vi "MoD Main-Optimize - HPLCv2 SnAr.vi"() -> ()   [LabVIEW 2015]
uses:
  <vilib>/silver_ctls/ArrayMatrixCluster/Real Matrix NI_Silver.ctl
  <vilib>/ni845x/ni845x.llb/ni845xControl.ctl
  <vilib>/MakerHub/LINX/Public/Peripherals/Analog/Analog Read 1 Chan.vi
  <vilib>/MakerHub/LINX/Public/Peripherals/Analog/Analog Read N Chans.vi
  <vilib>/MakerHub/LINX/Public/Peripherals/Digital/Digital Write 1 Chan.vi
  <vilib>/MakerHub/LINX/Private/Local IO/LinxAnalogRead.vi
  <vilib>/MakerHub/LINX/Public/Utilities/Check Channel.vi
  <vilib>/MakerHub/LINX/Public/Peripherals/Digital/Digital Write N Chans.vi
  <vilib>/MakerHub/LINX/Private/Local IO/LinxDigitalWrite.vi
  <vilib>/addons/control/pid/pid.llb/PID Control Input Filter (DBL).vi
  <vilib>/MakerHub/LINX/Private/Utilties/Generate Error.vi
  <vilib>/addons/control/pid/autopid.llb/PID Online Autotuning (Relay Feedback).vi
  <vilib>/Analysis/Matrix/Numeric/Conversions/Array To Matrix - RA2.vi
  <vilib>/ni845x/ni845x.llb/NI-845x Close Device Reference.vi
  <vilib>/addons/control/pid/NI_PID_autopid.lvlib
  <vilib>/addons/control/pid/NI_PID_pid.lvlib
  <vilib>/Analysis/Matrix/NI_Matrix.lvlib
  <vilib>/MakerHub/LINX/LMH-LINX.lvlib
  <instrlib>/Harvard Apparatus PHD Ultra Series/Harvard Apparatus PHD Ultra Series.lvlib
panel:
  out "running?":bool=TRUE
  out "new_reactor_volume":bool[](array[boolean])
  out "new_reactor_length":bool[](array[boolean])
  out "Phase_Sensor_voltage":dbl
  out "P_tot":dbl
  out "pause for ms":bool=TRUE
  out "stop_xl_write":bool=TRUE
  out "Num_exp_till_pause":i32
  out "Syringe_pump?":bool=TRUE
  out "System Error":bool=TRUE
  out "error out":errorcluster
  out "Pump setpoint(ul/min) 6":dbl format="%#_13g"
  out "Pump setpoint(ul/min) 5":dbl format="%#_13g"
  out "Pump setpoint(ul/min) 4":dbl format="%#_13g"
  out "Pump setpoint(ul/min) 3":dbl format="%#_13g"
  out "Pump setpoint(ul/min) 2":dbl format="%#_13g"
  out "Pump setpoint(ul/min) 1":dbl format="%#_13g"
  out "Volume (ul) 5":dbl format="%#_13g"
  out "Volume (ul) 4":dbl format="%#_13g"
  out "Volume (ul) 3":dbl format="%#_13g"
  out "Volume (ul) 2":dbl format="%#_13g"
  out "Volume (ul) 1":dbl format="%#_13g"
  in  "tau 5":dbl format="%#_13g"
  out "tau 4":dbl format="%#_13g"
  out "tau 3":dbl format="%#_13g"
  out "tau 2":dbl format="%#_13g"
  out "tau 1":dbl format="%#_13g"
  out "Reactor Length":dbl format="%#_13g"
  out "Flowrate Sensor 2":dbl format="%#_13g"
  out "Flowrate Sensor 1":dbl format="%#_13g"
  out "Pressure 2":dbl format="%#_13g"
  out "Pressure 1":dbl format="%#_13g"
  out "Temperature Control 5":bool=TRUE
  out "Temperature Control 4":bool=TRUE
  out "Temperature Control 3":bool=TRUE
  out "Temperature Control 2":bool=TRUE
  out "Temperature Control 1":bool=TRUE
  out "Temperature SP 5":dbl format="%#_g'C"
  out "Temperature SP 4":dbl format="%#_g'C"
  out "Temperature SP 3":dbl format="%#_g'C"
  out "Temperature SP 2":dbl format="%#_g'C"
  out "Temperature SP 1":dbl format="%#_g'C"
  in  "Bay Temperature 5":dbl
  in  "SSR Duration 5":dbl
  in  "SSR Duration 4":dbl
  in  "SSR Duration 3":dbl
  in  "SSR Duration 2":dbl
  in  "SSR Duration 1":dbl
  in  "Total Product Amount":dbl=1.0 format="%#_gml"
  out "Setup Error":bool=TRUE
  out "Error Message":string
  out "ID CTR":i32
  in  "Tab Control":T1(tab)
  out "Reagent pic 5":picture
  in  "reagent name 5":string
  out "Reagent Pic 4":picture
  in  "reagent name 4":string="DMF"
  out "Reagent Pic 3":picture
  in  "reagent  name 3":string="tributylamine"
  in  "Product name":string
  in  "reagent name 1":string="2-chloronitrobenzene"
  out "Reagent Pic 1":picture
  in  "Vr5":dbl format="%#_guL"
  in  "Vr4":dbl format="%#_guL"
  in  "Vr3":dbl format="%#_guL"
  in  "Vr2":dbl format="%#_guL"
  in  "Vr1":dbl format="%#_guL"
  in  "System decide help Button":bool
  in  "Reaction Scheme Confirm":bool
  in  "Synthesis Route Array":string[][](array[string])=[["2-chloronitrobenzene", "1.0", "PhB(OH)2", "", "", ""], ["1,2,3,4-tetrahydroquinoline", "1.0", "-", "-", "-", "-"], ["tributylamine", "1.0", "-", "-", "-", "-"], ["DMF", "8", "-", "-", "-", "-"]]
  in  "System decide help Button 2":bool
  out "Setup Confirm":bool=TRUE
  in  "BAY 1":u16(ring) items=["               Bypass", "         Heated Reactor", "    Small Heated Reator", "         Cooled Reactor", "      Packed Bed Reactor", "          Photo Reactor", "             Separator"]
  in  "BAY 5":u16(ring) items=["               Bypass", "         Heated Reactor", "    Small Heated Reactor", "         Cooled Reactor", "     Packed Bed Reactor", "         Photo Reactor", "             Separator"]
  in  "BAY 4":u16(ring)=1 items=["                Bypass", "         Heated Reactor", "    Small Heated Reactor", "         Cooled Reactor", "     Packed Bed Reactor", "         Photo Reactor", "             Separator"]
  in  "BAY 3":u16(ring) items=["               Bypass", "         Heated Reactor", "    Small Heated Reactor", "         Cooled Reactor", "     Packed Bed Reactor", "          Photo Reactor", "             Separator"]
  in  "BAY 2":u16(ring) items=["               Bypass", "         Heated Reactor", "    Small Heated Reactor", "         Cooled Reactor", "      Packed Bed Reactor", "          Photo Reactor", "             Separator"]
  out "Reagent Pic 2":picture
  out "Product Pic":picture
  in  "reagent name 2":string="1,2,3,4-tetrahydroquinoline"
  in  "reagent name 6":string
  out "Reagent Pic 6":picture
  in  "System Parameters Help Button":bool
  out "Setup Confirm 2":bool
  in  "System Parameters Confirm Button":bool
  in  "Bay Parameters":T2={"Bay 1 "={"Pump 1 Flowrate"=0.0, "optimize_temp"=FALSE, "optimize_tau"=TRUE, "Run at set flowrate"=FALSE, "Pump 2 Flowrate"=0.0, "Temperature Params"=[40.0, 100.0, 100.0], "pump params 1"=[21.0, 214.0, 325.0], "pump params 2"=[21.0, 214.0, 325.0], "Temperature"=0.0, "Run at set temperature"=FALSE}, "Bay 2 "={"Pump 3 Flowrate"=0.0, "optimize_temp"=FALSE, "optimize_tau"=FALSE, "Run at set flowrate"=TRUE, "Temperature Params"=[40.0, 100.0, 100.0], "Resisdence time params"=[65.0, 650.0, 650.0], "pump_at_ratio"=FALSE, "pump_num_ratio"=1.0, "Temperature"=0.0, "Run at set temperature"=FALSE}, "Bay 3 "={"Pump 4 Flowrate"=100.0, "optimize_temp"=FALSE, "optimize_tau"=TRUE, "Run at set flowrate"=FALSE, "Temperature Params"=[40.0, 100.0, 100.0], "Resisdence time params"=[21.0, 214.0, 0.0], "pump_at_ratio"=FALSE, "pump_num_ratio"=0.0, "Temperature "=0.0, "Run at set temperature"=FALSE}, "Bay 4 "={"Pump 5 Flowrate"=40.0, "Run at set flowrate"=FALSE, "optimize_temp"=TRUE, "optimize_tau"=FALSE, "Resisdence time params"=[0.0, 36.0, 225.0], "Temperature Params"=[40.0, 100.0, 80.0], "pump_at_ratio"=FALSE, "pump_num_ratio"=0.0, "Temperature"=0.0, "Run at set temperature"=FALSE}, "Bay 5 "={"Pump 6 Flowrate"=0.0, "Run at set flowrate"=FALSE, "optimize_temp"=FALSE, "optimize_tau"=FALSE, "Resisdence time params"=[0.0, 0.0, 0.0], "Temperature Params"=[0.0, 0.0, 0.0], "pump_at_ratio"=FALSE, "pump_num_ratio"=0.2, "Temperature"=0.0, "Run at set temperature"=FALSE}, "Excel File Name"="C:\\Users\\HPLC\\Dropbox (MIT)\\MoD Files\\Data\\SNAR_043017", "hplc File Name"="C:\\Chem32\\1\\Data\\MOD", "Matlab File"="C:\\Users\\HPLC\\Dropbox (MIT)\\MoD Files\\Data\\SNAR_043017", "Syringe for Pump 2?"=TRUE, "Num_conditons_per_wait"=1.0, "Continue from previous optimization?"=FALSE, "Total Number of Experiments 2"=33.0, "Hplc Wait time(min)"=14.0, "increas_decrease_hplc_peak"=FALSE, "Internal Standard?"=TRUE, "ISTD start"=10.0, "ISTD end"=14.0, "hplc_start"=2.3, "hplc_end"=2.8, "throughput_yield"=FALSE} {"Hplc Wait time(min)" format="%#_13g"; "Bay 5"."Temperature Params" format="%#_g'C"; "Bay 4"."Temperature Params" format="%#_g'C"; "Bay 3"."Temperature Params" format="%#_g'C"; "Bay 2"."Temperature Params" format="%#_g'C"; "Bay 1"."Temperature Params" format="%#_g'C"}
  out "System Confirm Not Clicked":string
  out "best_exp_num":dbl=1.0
  out "temperature_best":dbl[](array[numeric])
  out "Flowrates(ul/min)_best":dbl[](array[numeric])
  out "System Status":u16(ring)=2 caption="Sy" items=["System  Error", "System Running", "System Standby"]
  out "Current Experiment":dbl=1.0
  out "Total Number of Experiments":dbl=33.0
  out "Phase Sensor Chart":T3(graph)
  out "HPLC Analysis":bool
  out "Equlibrating Temperature":bool
  out "Flushing System":bool
  out "Calculate condition":bool
  out "Temperature 5":dbl format="%#_g'C"
  out "Temperature 4":dbl format="%#_g'C"
  out "Temperature 3":dbl format="%#_g'C"
  out "Temperature 2":dbl format="%#_g'C"
  out "Temperature 1":dbl format="%#_g'C"
  out "Flowrate Chart":T4(graph)
  out "Teperature Chart":T3(graph)
  out "Pump Setpoints Chart":T3(graph)
  out "Pressure Chart":T3(graph)
  out "Optimization_loop_index":i32
  out "curr_wait_time":dbl
  out "total_flush_time":dbl
  out "Temp SS? 5":bool=TRUE
  out "Temp SS? 4":bool=TRUE
  out "Temp SS? 3":bool=TRUE
  out "Temp SS? 2":bool=TRUE
  out "Temp SS? 1":bool=TRUE
  out "System Flushed?":bool
  out "stop_button clicked":bool
  out "experiment history":T5
  in  "Number of System Flushes per condtion":dbl=2.5
  in  "calculate volume 3":bool
  in  "calculate volume 2":bool
  in  "calculate volume 1":bool
  in  "calculate volume 4":bool
  in  "calculate volume 5":bool
  in  "Extra system dead volume":dbl format="%#_gul"
  in  "new reactor length? 1":bool
  in  "tube_length(in)":dbl[](array[numeric])=[188.0, 188.0, 10.0, 10.0, 10.0]
  out "Pause Before Analysis":bool
  out "Chiller COMM Port":bool
  out "Arduino COMM Port 2":bool
  out "Temperature Sensor COMM Port":bool
  out "Flow Rate":bool
  out "Pressure":bool
  out "Pump COMM Port":bool
  in  "COMM Port :: Milligat Pumps":refnum<visa-resource-name>="COM10"
  in  "Arduino COMM Port":refnum<visa-resource-name>="COM3"
  in  "Sample Valve COMM::Port":refnum<visa-resource-name>="COM6"
  in  "COMM Port:: Harvard Syringe Pump":refnum<visa-resource-name>="COM5"
  in  "tube_id(in)":enum16{".01", ".02", ".03", ".04"}[](array[ring])=[enum.".03", enum.".03", enum.".03", enum.".03", enum.".03"]
  out "Total System Resisdence Time(min)":dbl
  in  "Debug_run_button":bool
  in  "new reactor length? 2":bool
  in  "new reactor length? 3":bool
  in  "new reactor length? 4":bool
  in  "new reactor length? 5":bool
  in  "IR Sensor Device":T6="USB0::0x3923::0x7514::01B3FF21::RAW"
  out "Stop":bool=TRUE
  in  "Run_Stop_cluster":T7
  # "Molecules on Demand"
  # "Synthetic Route"
  # "5"
  # "6"
  # "4"
  # "Product"
  # "1"
  # "2"
  # "3"
  # "Reagent List"
  # "Concentration(M)"
  # "Molecule"
  # "1"
  # "1"
  # "2"
  # "2"
  # "3"
  # "3"
  # "4"
  # "4"
  # "5"
  # "6"
  # "5"
  # "6"
  # "Product"
  # "Reactor Volume:"
  # "Optimization Parameters"
  # "Pause after"
  # "Experiments"
  # "Optimize for"
  # "to"
  # "of HPLC Peak from"
  # "from"
  # "to"
  # "min"
  # "min"
  # "HPLC runtime"
  # "# Iterations"
  # "Reporting"
  # "Excel Output File Name"
  # "HPLC File Path"
  # "MATLAB File Path"
  # "Temperature"
  # "Flowrate(ul/min)"
  # "Lower Bound"
  # "Upper Bound"
  # "Optimize?"
  # "-or-"
  # "Run at"
  # "times incoming flow"
  # "Setpoint"
  # "Temperature"
  # "Flowrate(ul/min)"
  # "Lower Bound"
  # "Upper Bound"
  # "Optimize?"
  # "-or-"
  # "Run at"
  # "times incoming flow"
  # "Setpoint"
  # "Temperature"
  # "Flowrate(ul/min)"
  # "Lower Bound"
  # "Upper Bound"
  # "Optimize?"
  # "-or-"
  # "Run at"
  # "times incoming flow"
  # "Setpoint"
  # "Temperature"
  # "Flowrate 3 (ul/min)"
  # "Lower Bound"
  # "Upper Bound"
  # "Optimize?"
  # "-or-"
  # "Run at"
  # "times incoming flow"
  # "Setpoint"
  # "Temperature"
  # "Flowrate 1(ul/min)"
  # "Flowrate 2(ul/min)"
  # "Lower Bound"
  # "Upper Bound"
  # "Optimize?"
  # "Setpoint"
  # "Pressure (psi)"
  # "System Status"
  # "Temperature('C)"
  # "BAY"
  # "1"
  # "2"
  # "3"
  # "4"
  # "5"
  # "Pump Flowrate Setpoint(ul/min)"
  # "Flowrate (ul/min)"
  # "Phase Sensor"
  # "Current Experiment"
  # "Temperature('C)"
  # "Flowrate(ul/min)"
  # "Exp"
  # "Current Best Condition"
  # "Time to reach steady state:"
  # "Current Wait Time:"
  # "Experimental Steps"
  # "Calculated new conditions"
  # "Flushed System"
  # "Analyzed HPLC"
  # "Equilibrated Temperature"
  # "Tube Length (cm)"
  # "Bay"
  # "Tube ID (in)"
  # "Calculate Volume"
  # "Use new tube length"
  # "1."
  # "2."
  # "3."
  # "4."
  # "5."
  # "Reactor Lengths\n*Heated Reactor - 188cm * Small Reactor - 99cm * Bypass - 10cm * Separator - *"
  # "All Experimental Data"
  # "P1"
  # "P2"
  # "P3"
  # "P4"
  # "P5"
  # "P6"
  # "T1"
  # "T2"
  # "T3"
  # "T4"
  # "T5"
  # "Obj_fun"
  # "HPLC_Data"
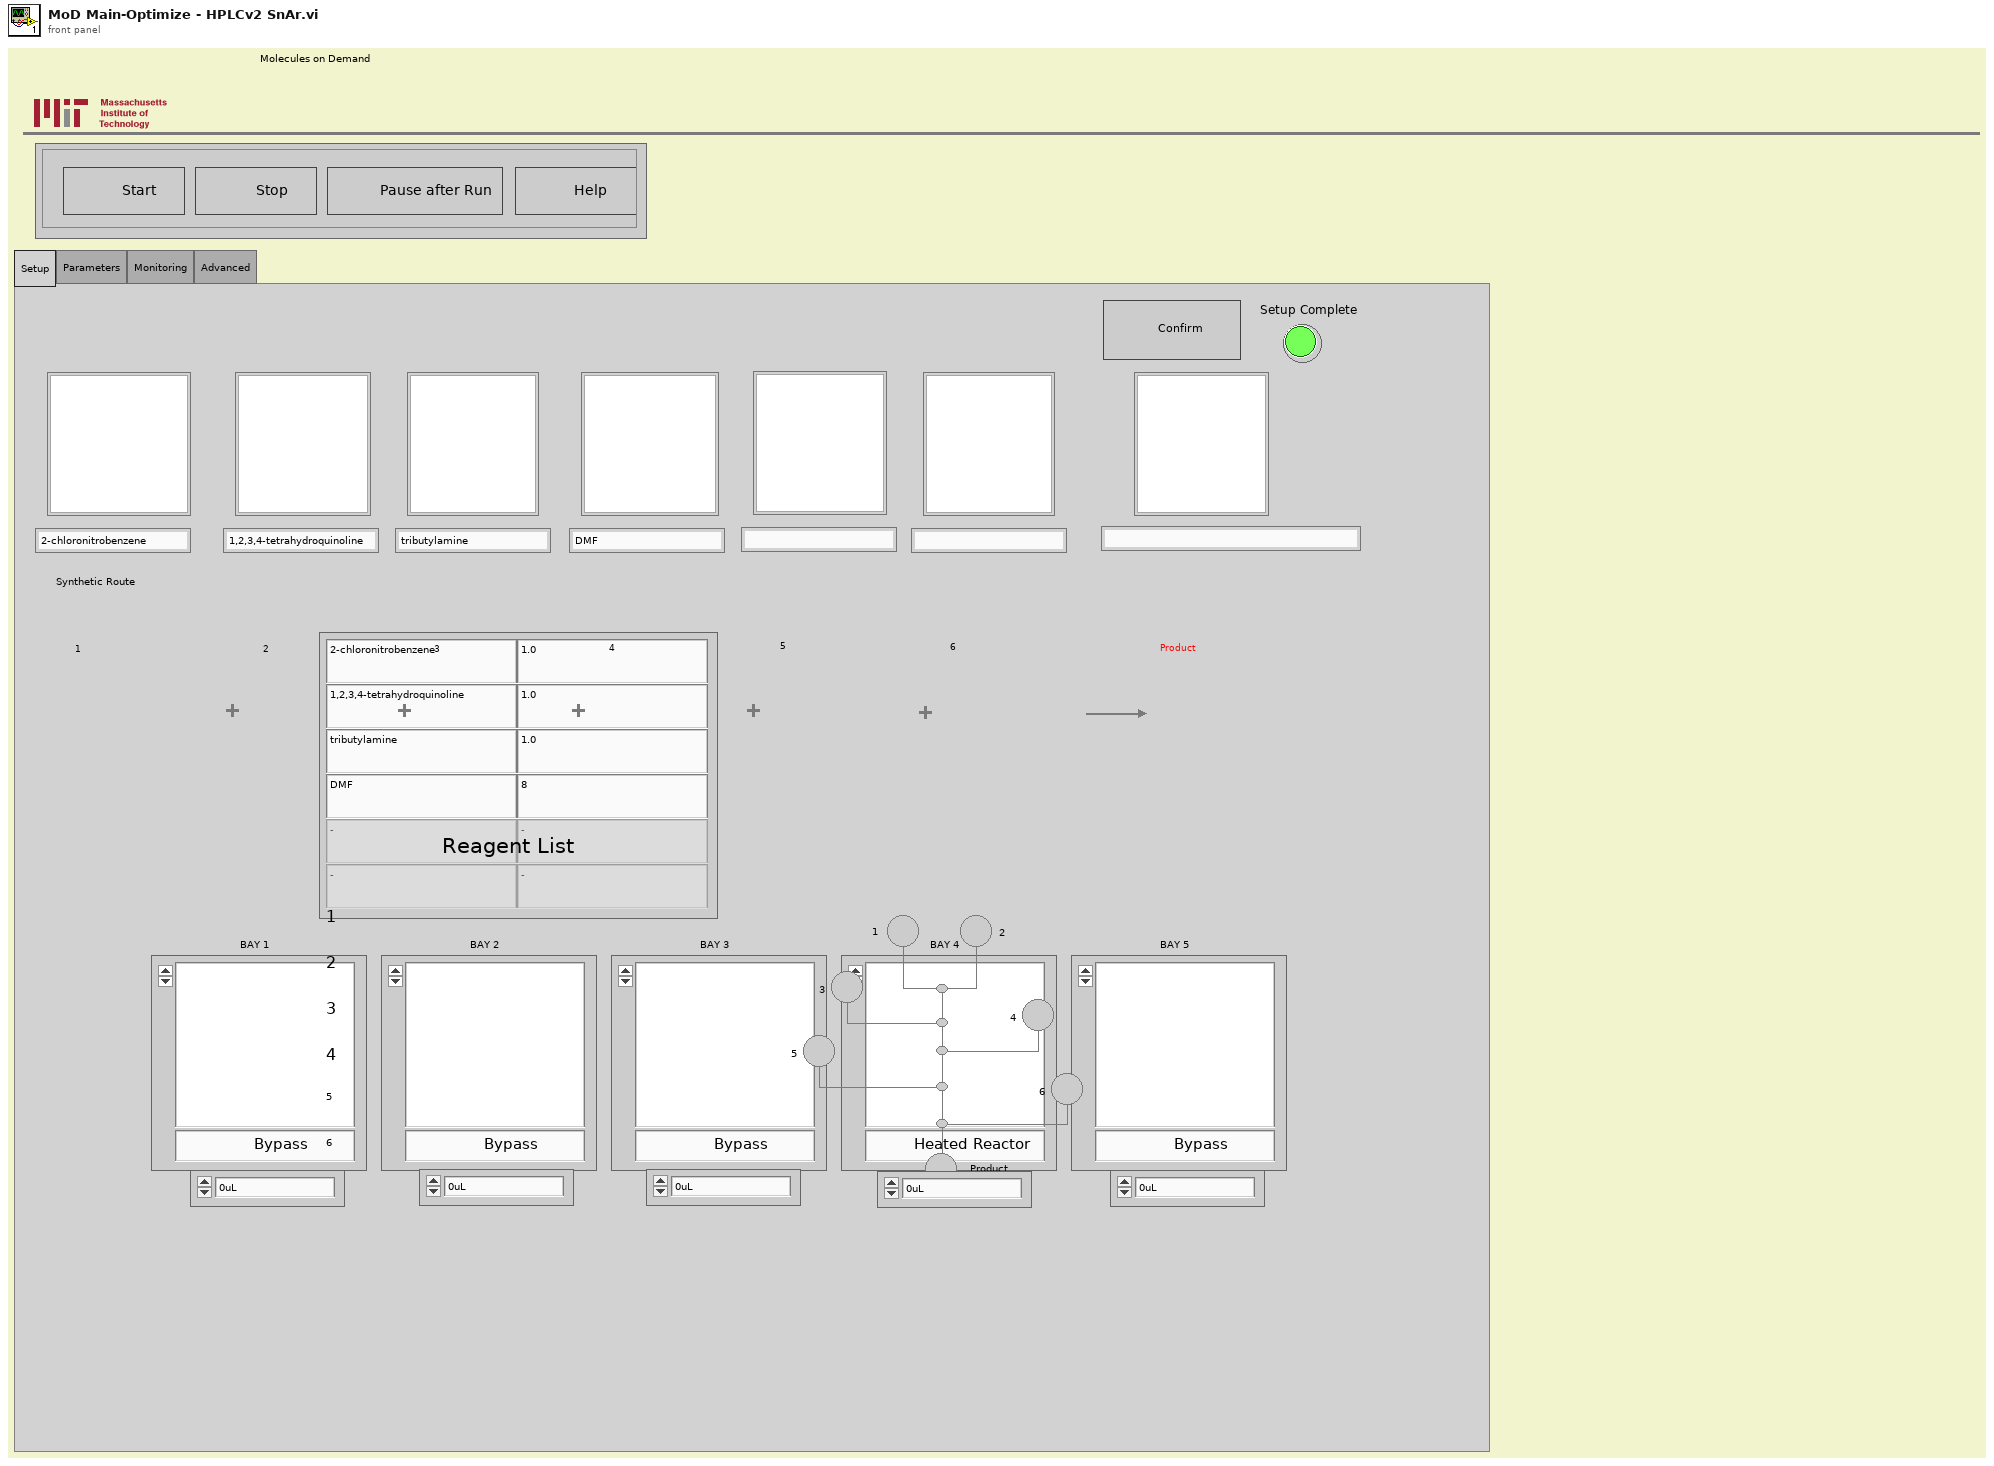
[diagram p1: front panel]
types:
  T1 = enum32{"Setup", "Parameters", "Monitoring", "Advanced"}
  T2 = cluster{"Bay 1 ":cluster{"Pump 1 Flowrate":dbl, "optimize_temp":bool, "optimize_tau":bool, "Run at set flowrate":bool, "Pump 2 Flowrate":dbl, "Temperature Params":dbl[], "pump params 1":dbl[], "pump params 2":dbl[], "Temperature":dbl, "Run at set temperature":bool}, "Bay 2 ":cluster{"Pump 3 Flowrate":dbl, "optimize_temp":bool, "optimize_tau":bool, "Run at set flowrate":bool, "Temperature Params":dbl[], "Resisdence time params":dbl[], "pump_at_ratio":bool, "pump_num_ratio":dbl, "Temperature":dbl, "Run at set temperature":bool}, "Bay 3 ":cluster{"Pump 4 Flowrate":dbl, "optimize_temp":bool, "optimize_tau":bool, "Run at set flowrate":bool, "Temperature Params":dbl[], "Resisdence time params":dbl[], "pump_at_ratio":bool, "pump_num_ratio":dbl, "Temperature ":dbl, "Run at set temperature":bool}, "Bay 4 ":cluster{"Pump 5 Flowrate":dbl, "Run at set flowrate":bool, "optimize_temp":bool, "optimize_tau":bool, "Resisdence time params":dbl[], "Temperature Params":dbl[], "pump_at_ratio":bool, "pump_num_ratio":dbl, "Temperature":dbl, "Run at set temperature":bool}, "Bay 5 ":cluster{"Pump 6 Flowrate":dbl, "Run at set flowrate":bool, "optimize_temp":bool, "optimize_tau":bool, "Resisdence time params":dbl[], "Temperature Params":dbl[], "pump_at_ratio":bool, "pump_num_ratio":dbl, "Temperature":dbl, "Run at set temperature":bool}, "Excel File Name":string, "hplc File Name":string, "Matlab File":string, "Syringe for Pump 2?":bool, "Num_conditons_per_wait":dbl, "Continue from previous optimization?":bool, "Total Number of Experiments 2":dbl, "Hplc Wait time(min)":dbl, "increas_decrease_hplc_peak":bool, "Internal Standard?":bool, "ISTD start":dbl, "ISTD end":dbl, "hplc_start":dbl, "hplc_end":dbl, "throughput_yield":bool}
  T3 = cluster{"[0]":dbl, "[1]":dbl, "[2]":dbl, "[3]":dbl, "[4]":dbl, "[5]":dbl, "[6]":dbl, "[7]":dbl, "[8]":dbl}
  T4 = cluster{"[0]":i32, "[1]":i32, "[2]":i32, "[3]":i32, "[4]":i32, "[5]":i32, "[6]":i32, "[7]":i32, "[8]":i32}
  T5 = typedef "Real Matrix NI_Silver.ctl" = dbl[][]
  T6 = typedef "ni845xControl.ctl" = refnum<k21>
  T7 = cluster{"Stop":bool, "Run":bool, "Stop Run Button":bool, "Help Button":bool}
  T8 = cluster{"Proportional gain Kc":dbl, "Integral time Ti (sec)":dbl, "Derivative time Ti (sec)":dbl}
  T9 = cluster{"type of controller":enum16{"P", "PI", "PID"}, "relay cycles":i32, "relay amplitude":dbl, "control specifications":enum16{"Fast", "Normal", "Slow"}, "PV noise level":dbl}
  T10 = typedef "LMH-LINX.lvlib/LINX Ref.ctl" = cluster{"IO":T11, "Interface":T12, "LINX Device Config":T13}
  T11 = typedef "LMH-LINX.lvlib/Platform.ctl" = enum16{"Remote", "Local"}
  T12 = typedef "LMH-LINX.lvlib/Interface.ctl" = enum16{"Serial", "TCP"}
  T13 = typedef "LMH-LINX.lvlib/Device.lvlib/LINX Device Config.ctl" = cluster{"Interface":T12, "COM Port":refnum<visa-resource-name>, "TCP Configuration":T14, "Device Family":u8, "Device ID":u8, "Device Name":string, "TCP Ref":refnum<k5>, "Channels":T15}
  T14 = typedef "LMH-LINX.lvlib/Device.lvlib/TCP Config.ctl" = cluster{"IP Address":string, "Port":u16}
  T15 = typedef "LMH-LINX.lvlib/Channels.ctl" = cluster{"DI":u8[], "DO":u8[], "AI":u8[], "AO":u8[], "PWM":u8[], "QE":u8[], "UART":u8[], "I2C 2":u8[], "SPI":u8[], "CAN":u8[], "Servo":u8[], "AI Ref (V)":dbl, "AI Resolution (Bits)":u8, "AO Ref (V)":dbl, "AO Resolution (Bits)":u8}
  T16 = typedef "imagedata.ctl" = cluster{"image type":i32, "image depth":i32, "image":u8[], "mask":u8[], "colors":u32[], "Rectangle":cluster{"left":i16, "top":i16, "right":i16, "bottom":i16}}
  T17 = cluster{"proportional gain (Kc)":dbl, "integral time (Ti, min)":dbl, "derivative time (Td, min)":dbl}
  T18 = typedef "NI_Matrix.lvlib/RealMatrix.ctl" = dbl[][]
  T19 = enum16{"Left Button", "Center Button", "Right Button", "Window Close"}
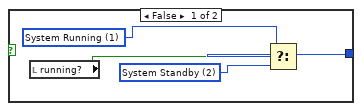
[diagram p3: hidden frame]
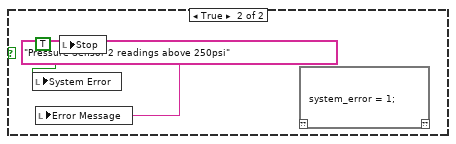
[diagram p4: hidden frame]
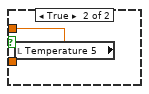
[diagram p6: hidden frame]
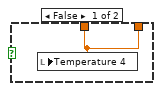
[diagram p7: hidden frame]
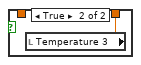
[diagram p8: hidden frame]
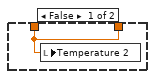
[diagram p9: hidden frame]
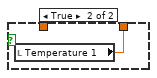
[diagram p10: hidden frame]
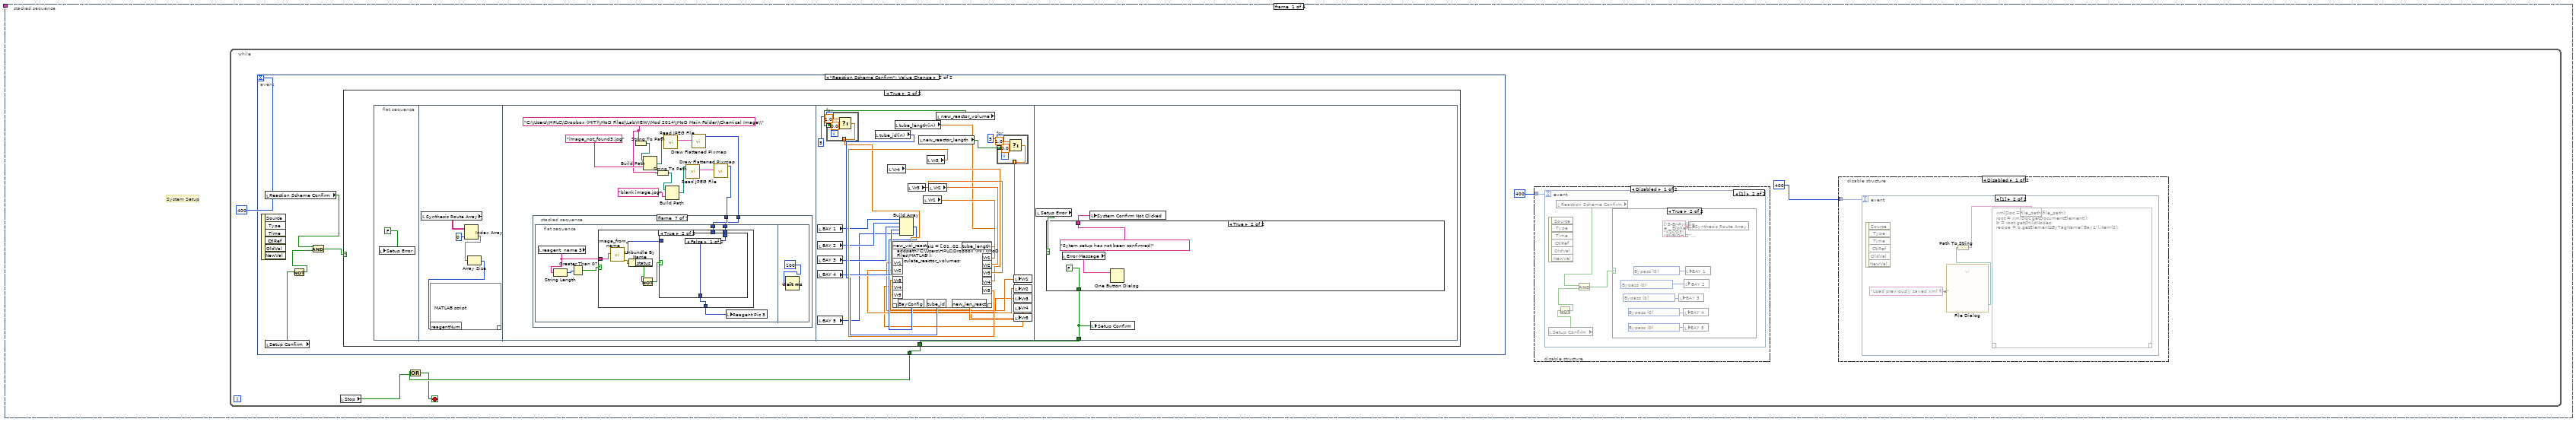
[diagram p11: hidden frame]
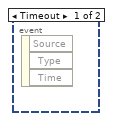
[diagram p12: hidden frame]
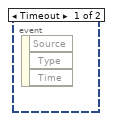
[diagram p14: hidden frame]
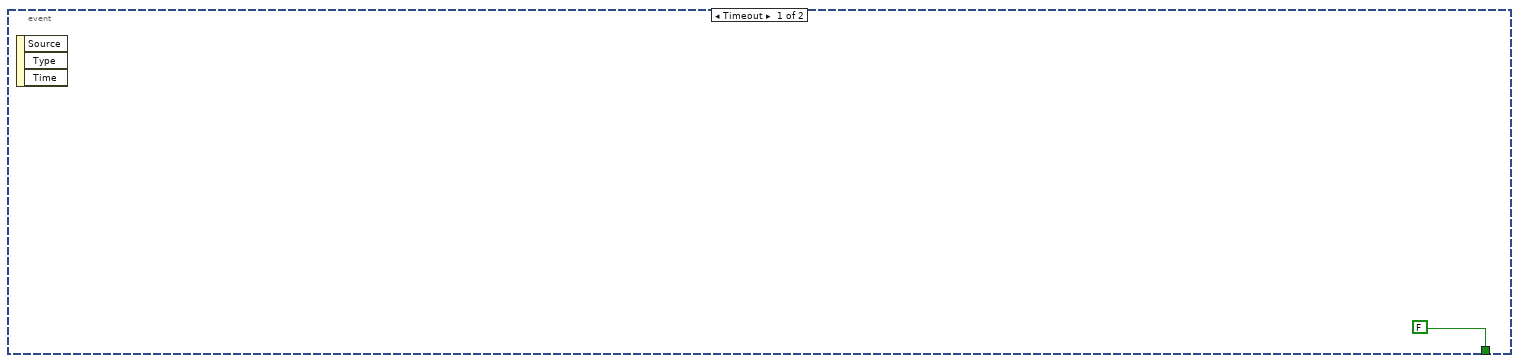
[diagram p17: hidden frame]
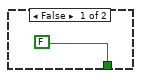
[diagram p18: hidden frame]
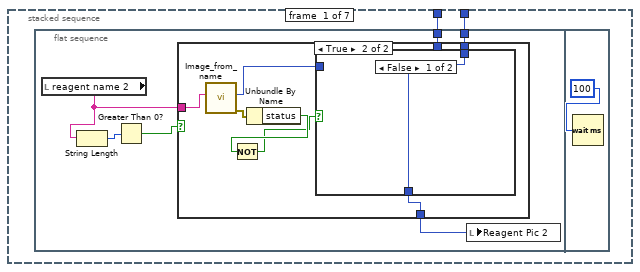
[diagram p19: hidden frame]
diagram:
  # "Assume User always uses the first bay first"
  n1 = flat-sequence {
    tunnel: ["COMM Port :: Milligat Pumps"] -> w9
    tunnel: ["Arduino COMM Port"] -> w8
    tunnel: ["COMM Port:: Harvard Syringe Pump"] -> w5
    tunnel: ["Bay Parameters"] -> w4
    tunnel: [w59] -> w10
    tunnel: w9 -> [w59]
    tunnel: w8 -> [w47]
    tunnel: [w53] -> w7
    tunnel: [w51] -> w6
    tunnel: w5 -> [w51]
    tunnel: w4 -> [w49]
    tunnel: [w46] -> w3
    tunnel: w10 -> [w65]
    tunnel: w7 -> [w64]
    tunnel: w6 -> [w62]
    tunnel: w3 -> [w60]
    tunnel: [w60] -> w1
    tunnel: [w1335] -> w2
    tunnel: w1 -> [w1335]
    tunnel: w2 -> [w1336]
    frame #0 {
      w35 = FALSE ("Equlibrating Temperature")
      n2 = script code="TempArr1=[23 23 23 23 23 23 23 23 23 23]';\nTempArr2=[23 23 23 23 23 23 23 23 23 23]';\nTempArr3=[23 23 23 23 23 23 23 23 23 23]';\nTempArr4=[23 23 23 23 23 23 23 23 23 23]';\nTempArr5=[23 23 23 23 23 23 23 23 23 23]';\ntemp_error1 =0;\ntemp_error2 =0;\ntemp_error3 =0;\ntemp_error4 =0;\ntemp_error5 =0;\ntemp_check1 = 0;\ntemp_check2 = 0;\ntemp_check3 = 0;\ntemp_check4 = 0;\ntemp_check5 = 0;\nT1=23;\nT2=23;\nT3=23;\nT4=23;\nT5=23;"() -> ()  [unwired: 1 in, 1 out]
      n3 = Build Array("calculate volume 1", "calculate volume 2", "calculate volume 3", "calculate volume 4", "calculate volume 5") -> (→"new_reactor_volume":bool[])
      n4 = Build Array("new reactor length? 1", "new reactor length? 2", "new reactor length? 3", "new reactor length? 4", "new reactor length? 5") -> (→"new_reactor_length":bool[])
      "Stop" <- FALSE ("Stop")
      "ID CTR" <- 0
      "Setup Confirm" <- FALSE ("Setup Confirm")
      "Error Message" <- "System shutdown sucessfully. No errors to report." ("Error Message")
      "Setup Error" <- FALSE ("Setup Error")
      "Reactor Length" <- 10.5
      "System Error" <- FALSE ("System Error")
      "Num_exp_till_pause" <- 0 ("Num_exp_till_pause")
      "Equlibrating Temperature" <- w35
      "Calculate condition" <- w35
      "Flushing System" <- w35
      "HPLC Analysis" <- w35
      "stop_xl_write" <- FALSE ("stop_xl_write")
      "Pump setpoint(ul/min) 1" <- 0.0 ("Pump setpoint(ul/min) 1")
      "Pump setpoint(ul/min) 2" <- 0.0 ("Pump setpoint(ul/min) 2")
      "Pump setpoint(ul/min) 4" <- 0.0 ("Pump setpoint(ul/min) 4")
      "Pump setpoint(ul/min) 6" <- 0.0 ("Pump setpoint(ul/min) 6")
      "Pump setpoint(ul/min) 3" <- 0.0 ("Pump setpoint(ul/min) 3")
      "Pump setpoint(ul/min) 5" <- 0.0 ("Pump setpoint(ul/min) 5")
      "pause for ms" <- FALSE ("pause for ms")
      "Setup Confirm 2" <- FALSE ("Setup Confirm 2")
      "running?" <- FALSE ("running?")
    }
    frame #1 {
      w48 = FALSE
      w58 = 23
      (unwired) path "C:/Users/User1/Documents/Lab/MoD/Images"
      n5 = disable-structure shown="Disabled" {
        frame Disabled {
          n6 = local read "BAY 2"() -> ()  [unwired: 1 out]
          n7 = local read "BAY 3"() -> ()  [unwired: 1 out]
          n8 = local read "BAY 4"() -> ()  [unwired: 1 out]
          n9 = local read "BAY 5"() -> ()  [unwired: 1 out]
          n10 = local read "BAY 1"() -> ()  [unwired: 1 out]
        }
        frame Enabled {
        }
      }
      n11 = local write "Debug_run_button"(TRUE) -> ()
      n12 = call <vilib>:"Initialize.vi"("Serial Port"=w47) -> ("LINX Resource"=w46:T10)  [unwired: 8 in, 2 out]
      n13 = local write "System Parameters Confirm Button"(w48) -> ()
      n14 = local write "Setup Confirm 2"(w48) -> ()
      n15 = Unbundle By Name(w49) -> ("Syringe for Pump 2?"=→"Syringe_pump?":bool)
      n16 = local write "Temperature 1"(w58) -> ()
      n17 = local write "Temperature 2"(w58) -> ()
      n18 = local write "Temperature 3"(w58) -> ()
      n19 = local write "Temperature 4"(w58) -> ()
      n20 = local write "Temperature 5"(w58) -> ()
      n21 = local write "Temperature SP 1"(w58) -> ()
      n22 = local write "Temperature SP 2"(w58) -> ()
      n23 = local write "Temperature SP 3"(w58) -> ()
      n24 = local write "Temperature SP 4"(w58) -> ()
      n25 = local write "Temperature SP 5"(w58) -> ()
      n26 = Current VI's Path() -> (path=w57:path)
      n27 = Strip Path(path=w57) -> (stripped path=w55:path)  [unwired: 1 out]
      n28 = Strip Path(path=w55) -> (stripped path=w54:path)  [unwired: 1 out]
      n29 = Build Path(base path=w54, name or relative path="MATLAB") -> (appended path=w53:path)
    }
    frame #2 {
      # "Main Help Dialog Popup"
      n30 = while {
        stop <- w1329 stop-if-true
        n31 = event shown="[6] \"Run_Stop_cluster.Run\": Value Change" {
          selector: _ -> [_ _ _ _ _ _ _]
          dyn-events: _ -> [_ _ _ _ _ _ _]
          timeout: 100 -> [_ _ _ _ _ _ _]
          event Timeout {
            n32 = event-data() -> ()  [unwired: 1 in, 3 out]
          }
          event "Run_Stop_cluster.Help Button": Value Change {
            n33 = local read "Run_Stop_cluster"() -> (w1332:T7)
            n34 = event-data() -> ()  [unwired: 1 in, 4 out]
            n35 = Unbundle By Name(w1332) -> ("Help Button"=w1331:bool)
            n36 = case shown="True" w1331 {
              frame False {
              }
              frame True {
                n37 = call "help.vi"() -> ()  [unwired: 11 in]
              }
            }
          }
          event "System decide help Button": Value Change {
            n38 = event-data() -> ()  [unwired: 1 in, 5 out]
            n39 = call "help_synthesis_man-auto_instructions.vi"() -> ()  [unwired: 12 in]
          }
          event "System Parameters Help Button": Value Change {
            n40 = event-data() -> ()  [unwired: 1 in, 5 out]
            n41 = call "help_parameters_setup.vi"() -> ()  [unwired: 12 in]
          }
          event "System decide help Button 2": Value Change {
            n42 = event-data() -> ()  [unwired: 1 in, 5 out]
            n43 = call "help_synthesis_route_instructions.vi"() -> ()  [unwired: 12 in]
          }
          event "Run_Stop_cluster.Stop": Value Change {
            n44 = event-data() -> ()  [unwired: 1 in, 5 out]
            n45 = local write "Stop"(TRUE) -> ()
          }
          event "Run_Stop_cluster.Run": Value Change {
            n46 = event-data() -> ()  [unwired: 1 in, 5 out]
            n47 = local write "running?"(TRUE) -> ()
          }
        }
        n48 = local read "Stop"() -> (w1329:bool)
      }
      n49 = stacked-sequence {
        tunnel: w65 -> [_ _ _ _]
        tunnel: w64 -> [_ w424 _ _]
        tunnel: w62 -> [_ _ _ w587]
        tunnel: w60 -> [_ _ _ w585]
        frame #0 {
          # "System Setup"
          n50 = while {
            stop <- w199 stop-if-true
            n51 = event shown="[1] \"Reaction Scheme Confirm\": Value Change" {
              selector: _ -> [_ _]
              dyn-events: _ -> [_ _]
              timeout: 400 -> [_ _]
              tunnel: [FALSE w219] -> w201
              event Timeout {
                n52 = event-data() -> ()  [unwired: 1 in, 3 out]
              }
              event "Reaction Scheme Confirm": Value Change {
                n53 = event-data() -> ()  [unwired: 1 in, 6 out]
                n54 = local read "Reaction Scheme Confirm"() -> (w223:bool)
                n55 = local read "Setup Confirm"() -> (w221:bool)
                n56 = Not(x=w221) -> (.not. x?=w220:bool)
                n57 = And(x=w223, y=w220) -> (x .and. y?=w222:bool)
                n58 = case shown="True" w222 {
                  tunnel: [FALSE w225] -> w219
                  frame False {
                  }
                  frame True {
                    n59 = flat-sequence {
                      tunnel: [w414] -> w225
                      frame #0 {
                        n60 = local write "Setup Error"(FALSE) -> ()
                      }
                      frame #1 {
                        n61 = local read "Synthesis Route Array"() -> (w229:string[][])
                        n62 = Index Array(array=w229, index (col)=0 ("disabled index (col)")) -> (element=w227:string[])  [unwired: 1 in]
                        n63 = Array Size(array=w227) -> (size(s)=w230:i32)
                        n64 = script code="MATLAB script"("reagentNum"=w230) -> ()  [unwired: 1 in, 1 out]
                      }
                      frame #2 {
                        w233 = "C:\\Users\\HPLC\\Dropbox (MIT)\\MoD Files\\LabVIEW\\Mod 2014\\MoD Main Folder\\Chemical Image\\" ("string")
                        n65 = String To Path(string=w233) -> (path=w239:path)
                        n66 = Build Path(base path=w239, name or relative path="image_not_found3.jpg") -> (appended path=w238:path)
                        n67 = String To Path(string=w233) -> (path=w236:path)
                        n68 = call <vilib>:"Read JPEG File.vi"("path to JPEG file"=w238) -> ("image data"=w241:T16)  [unwired: 1 in, 9 out]
                        n69 = Build Path(base path=w236, name or relative path="blank image.jpg") -> (appended path=w234:path)
                        n70 = call <vilib>:"Read JPEG File.vi"("path to JPEG file"=w234) -> ("image data"=w237:T16)  [unwired: 1 in, 9 out]
                        n71 = call <vilib>:"Draw Flattened Pixmap.vi"("image data"=w241) -> ("new picture"=w232:picture)  [unwired: 3 in, 5 out]
                        n72 = call <vilib>:"Draw Flattened Pixmap.vi"("image data"=w237) -> ("new picture"=w231:picture)  [unwired: 3 in, 5 out]
                        n73 = stacked-sequence {
                          tunnel: w232 -> [w243 w263 w283 w303 w323 w342 w362]
                          tunnel: w231 -> [w242 w262 w282 w302 w322 w343 w363]
                          frame #0 {
                            n74 = flat-sequence {
                              tunnel: w243 -> [w249]
                              tunnel: w242 -> [w247]
                              frame #0 {
                                n75 = local read "reagent name 2"() -> (w245:string)
                                n76 = String Length(string=w245) -> (length=w248:i32)
                                n77 = Greater Than 0?(x=w248) -> (x > 0?=w246:bool)
                                n78 = case shown="True" w246 {
                                tunnel: w249 -> [_ w255]
                                tunnel: w247 -> [w250 _]
                                tunnel: [w250 w254] -> w244
                                tunnel: w245 -> [_ w253]
                                frame False {
                                }
                                frame True {
                                n79 = call "Image_from_name.vi"("Chemical Name"=w253) -> ("error out"=w256:errorcluster, "Downloaded Picture"=w257:picture)  [unwired: 8 in, 1 out]
                                n80 = Unbundle By Name(w256) -> ("status"=w252:bool)
                                n81 = Not(x=w252) -> (.not. x?=w251:bool)
                                n82 = case shown="False" w251 {
                                tunnel: w257 -> [_ w260]
                                tunnel: [w258 w259] -> w254
                                tunnel: w255 -> [w258 _]
                                frame False {
                                }
                                frame True {
                                n83 = call <vilib>:"Draw Flattened Pixmap.vi"("picture"=w260) -> ("new picture"=w259:picture)  [unwired: 8 in]
                                }
                                }
                                }
                                }
                                n84 = local write "Reagent Pic 2"(w244) -> ()
                              }
                              frame #1 {
                                n85 = Wait (ms)(milliseconds to wait=100) -> ()  [unwired: 1 out]
                              }
                            }
                          }
                          frame #1 {
                            n86 = flat-sequence {
                              tunnel: w263 -> [w269]
                              tunnel: w262 -> [w267]
                              frame #0 {
                                n87 = local read "reagent name 1"() -> (w264:string)
                                n88 = String Length(string=w264) -> (length=w268:i32)
                                n89 = Greater Than 0?(x=w268) -> (x > 0?=w266:bool)
                                n90 = case shown="True" w266 {
                                tunnel: w269 -> [_ w275]
                                tunnel: w267 -> [w270 _]
                                tunnel: [w270 w274] -> w265
                                tunnel: w264 -> [_ w273]
                                frame False {
                                }
                                frame True {
                                n91 = call "Image_from_name.vi"("Chemical Name"=w273) -> ("error out"=w276:errorcluster, "Downloaded Picture"=w277:picture)  [unwired: 8 in, 1 out]
                                n92 = Unbundle By Name(w276) -> ("status"=w272:bool)
                                n93 = Not(x=w272) -> (.not. x?=w271:bool)
                                n94 = case shown="True" w271 {
                                tunnel: w277 -> [_ w280]
                                tunnel: [w278 w279] -> w274
                                tunnel: w275 -> [w278 _]
                                frame False {
                                }
                                frame True {
                                n95 = call <vilib>:"Draw Flattened Pixmap.vi"("picture"=w280) -> ("new picture"=w279:picture)  [unwired: 8 in]
                                }
                                }
                                }
                                }
                                n96 = local write "Reagent Pic 1"(w265) -> ()
                              }
                              frame #1 {
                                n97 = Wait (ms)(milliseconds to wait=100) -> ()  [unwired: 1 out]
                              }
                            }
                          }
                          frame #2 {
                            n98 = flat-sequence {
                              tunnel: w283 -> [w289]
                              tunnel: w282 -> [w287]
                              frame #0 {
                                n99 = local read "Product name"() -> (w284:string)
                                n100 = String Length(string=w284) -> (length=w288:i32)
                                n101 = Greater Than 0?(x=w288) -> (x > 0?=w286:bool)
                                n102 = case shown="True" w286 {
                                tunnel: w289 -> [_ w295]
                                tunnel: w287 -> [w290 _]
                                tunnel: [w290 w294] -> w285
                                tunnel: w284 -> [_ w293]
                                frame False {
                                }
                                frame True {
                                n103 = call "Image_from_name.vi"("Chemical Name"=w293) -> ("error out"=w296:errorcluster, "Downloaded Picture"=w297:picture)  [unwired: 8 in, 1 out]
                                n104 = Unbundle By Name(w296) -> ("status"=w291:bool)
                                n105 = Not(x=w291) -> (.not. x?=w292:bool)
                                n106 = case shown="False" w292 {
                                tunnel: w297 -> [_ w300]
                                tunnel: [w298 w299] -> w294
                                tunnel: w295 -> [w298 _]
                                frame False {
                                }
                                frame True {
                                n107 = call <vilib>:"Draw Flattened Pixmap.vi"("picture"=w300) -> ("new picture"=w299:picture)  [unwired: 8 in]
                                }
                                }
                                }
                                }
                                n108 = local write "Product Pic"(w285) -> ()
                              }
                              frame #1 {
                                n109 = Wait (ms)(milliseconds to wait=100) -> ()  [unwired: 1 out]
                              }
                            }
                          }
                          frame #3 {
                            n110 = flat-sequence {
                              tunnel: w303 -> [w309]
                              tunnel: w302 -> [w307]
                              frame #0 {
                                n111 = local read "reagent name 6"() -> (w304:string)
                                n112 = String Length(string=w304) -> (length=w308:i32)
                                n113 = Greater Than 0?(x=w308) -> (x > 0?=w306:bool)
                                n114 = case shown="True" w306 {
                                tunnel: w309 -> [_ w315]
                                tunnel: w307 -> [w310 _]
                                tunnel: [w310 w314] -> w305
                                tunnel: w304 -> [_ w313]
                                frame False {
                                }
                                frame True {
                                n115 = call "Image_from_name.vi"("Chemical Name"=w313) -> ("error out"=w316:errorcluster, "Downloaded Picture"=w317:picture)  [unwired: 8 in, 1 out]
                                n116 = Unbundle By Name(w316) -> ("status"=w311:bool)
                                n117 = Not(x=w311) -> (.not. x?=w312:bool)
                                n118 = case shown="False" w312 {
                                tunnel: w317 -> [_ w320]
                                tunnel: [w318 w319] -> w314
                                tunnel: w315 -> [w318 _]
                                frame False {
                                }
                                frame True {
                                n119 = call <vilib>:"Draw Flattened Pixmap.vi"("picture"=w320) -> ("new picture"=w319:picture)  [unwired: 8 in]
                                }
                                }
                                }
                                }
                                n120 = local write "Reagent Pic 6"(w305) -> ()
                              }
                              frame #1 {
                                n121 = Wait (ms)(milliseconds to wait=100) -> ()  [unwired: 1 out]
                              }
                            }
                          }
                          frame #4 {
                            n122 = flat-sequence {
                              tunnel: w323 -> [w329]
                              tunnel: w322 -> [w327]
                              frame #0 {
                                n123 = local read "reagent name 5"() -> (w324:string)
                                n124 = String Length(string=w324) -> (length=w328:i32)
                                n125 = Greater Than 0?(x=w328) -> (x > 0?=w326:bool)
                                n126 = case shown="True" w326 {
                                tunnel: w329 -> [_ w335]
                                tunnel: w327 -> [w330 _]
                                tunnel: [w330 w334] -> w325
                                tunnel: w324 -> [_ w333]
                                frame False {
                                }
                                frame True {
                                n127 = call "Image_from_name.vi"("Chemical Name"=w333) -> ("error out"=w336:errorcluster, "Downloaded Picture"=w337:picture)  [unwired: 8 in, 1 out]
                                n128 = Unbundle By Name(w336) -> ("status"=w331:bool)
                                n129 = Not(x=w331) -> (.not. x?=w332:bool)
                                n130 = case shown="False" w332 {
                                tunnel: w337 -> [_ w340]
                                tunnel: [w338 w339] -> w334
                                tunnel: w335 -> [w338 _]
                                frame False {
                                }
                                frame True {
                                n131 = call <vilib>:"Draw Flattened Pixmap.vi"("picture"=w340) -> ("new picture"=w339:picture)  [unwired: 8 in]
                                }
                                }
                                }
                                }
                                n132 = local write "Reagent pic 5"(w325) -> ()
                              }
                              frame #1 {
                                n133 = Wait (ms)(milliseconds to wait=100) -> ()  [unwired: 1 out]
                              }
                            }
                          }
                          frame #5 {
                            n134 = flat-sequence {
                              tunnel: w343 -> [w347]
                              tunnel: w342 -> [w346]
                              frame #0 {
                                n135 = local read "reagent name 4"() -> (w344:string)
                                n136 = String Length(string=w344) -> (length=w349:i32)
                                n137 = Greater Than 0?(x=w349) -> (x > 0?=w348:bool)
                                n138 = case shown="True" w348 {
                                tunnel: w346 -> [_ w355]
                                tunnel: w347 -> [w350 _]
                                tunnel: [w350 w354] -> w345
                                tunnel: w344 -> [_ w353]
                                frame False {
                                }
                                frame True {
                                n139 = call "Image_from_name.vi"("Chemical Name"=w353) -> ("error out"=w356:errorcluster, "Downloaded Picture"=w357:picture)  [unwired: 8 in, 1 out]
                                n140 = Unbundle By Name(w356) -> ("status"=w351:bool)
                                n141 = Not(x=w351) -> (.not. x?=w352:bool)
                                n142 = case shown="False" w352 {
                                tunnel: w357 -> [_ w360]
                                tunnel: [w358 w359] -> w354
                                tunnel: w355 -> [w358 _]
                                frame False {
                                }
                                frame True {
                                n143 = call <vilib>:"Draw Flattened Pixmap.vi"("picture"=w360) -> ("new picture"=w359:picture)  [unwired: 8 in]
                                }
                                }
                                }
                                }
                                n144 = local write "Reagent Pic 4"(w345) -> ()
                              }
                              frame #1 {
                                n145 = Wait (ms)(milliseconds to wait=100) -> ()  [unwired: 1 out]
                              }
                            }
                          }
                          frame #6 {
                            n146 = flat-sequence {
                              tunnel: w363 -> [w367]
                              tunnel: w362 -> [w366]
                              frame #0 {
                                n147 = local read "reagent  name 3"() -> (w364:string)
                                n148 = String Length(string=w364) -> (length=w369:i32)
                                n149 = Greater Than 0?(x=w369) -> (x > 0?=w368:bool)
                                n150 = case shown="True" w368 {
                                tunnel: w366 -> [_ w375]
                                tunnel: w367 -> [w370 _]
                                tunnel: [w370 w374] -> w365
                                tunnel: w364 -> [_ w373]
                                frame False {
                                }
                                frame True {
                                n151 = call "Image_from_name.vi"("Chemical Name"=w373) -> ("error out"=w376:errorcluster, "Downloaded Picture"=w377:picture)  [unwired: 8 in, 1 out]
                                n152 = Unbundle By Name(w376) -> ("status"=w371:bool)
                                n153 = Not(x=w371) -> (.not. x?=w372:bool)
                                n154 = case shown="False" w372 {
                                tunnel: w377 -> [_ w380]
                                tunnel: [w378 w379] -> w374
                                tunnel: w375 -> [w378 _]
                                frame False {
                                }
                                frame True {
                                n155 = call <vilib>:"Draw Flattened Pixmap.vi"("picture"=w380) -> ("new picture"=w379:picture)  [unwired: 8 in]
                                }
                                }
                                }
                                }
                                n156 = local write "Reagent Pic 3"(w365) -> ()
                              }
                              frame #1 {
                                n157 = Wait (ms)(milliseconds to wait=100) -> ()  [unwired: 1 out]
                              }
                            }
                          }
                        }
                      }
                      frame #3 {
                        n158 = local read "BAY 1"() -> (w392:u16)
                        n159 = local read "BAY 2"() -> (w391:u16)
                        n160 = local read "BAY 3"() -> (w390:u16)
                        n161 = local read "BAY 4"() -> (w389:u16)
                        n162 = local read "BAY 5"() -> (w388:u16)
                        n163 = local read "tube_id(in)"() -> (w399:enum16{".01", ".02", ".03", ".04"}[])
                        n164 = local read "Vr4"() -> (w402:dbl)
                        n165 = local read "tube_length(in)"() -> (w400:dbl[])
                        n166 = Build Array(w392, w391, w390, w389, w388) -> (w387:u16[])
                        n167 = local read "Vr3"() -> (w403:dbl)
                        n168 = local read "new_reactor_length"() -> (w397:bool[])
                        n169 = local read "Vr1"() -> (w405:dbl)
                        n170 = local read "Vr5"() -> (w401:dbl)
                        n171 = local read "Vr2"() -> (w404:dbl)
                        n172 = local read "new_reactor_volume"() -> (w395:bool[])
                        n173 = for {
                          N: 5 -> [_]
                          tunnel: w395 -> [w409] mode=indexing
                          tunnel: [w406] -> w393 mode=indexing
                          n174 = Select(t=1.0, s=w409, f=0.0) -> (s? t:f=w406:dbl)
                        }
                        n175 = for {
                          N: 5 -> [_]
                          tunnel: w397 -> [w413] mode=indexing
                          tunnel: [w410] -> w396 mode=indexing
                          n176 = Select(t=1.0, s=w413, f=0.0) -> (s? t:f=w410:dbl)
                        }
                        n177 = script code="tube_diameters = [.01,.02,.03,.04];\naddpath('C:\\Users\\HPLC\\Dropbox (MIT)\\MoD Files\\MATLAB');\ncalculate_reactor_volumes;"("BayConfig"=w387, "Vr1"=w405, "Vr2"=w404, "Vr3"=w403, "Vr4"=w402, "Vr5"=w401, "tube_length"=w400, "tube_id"=w399, "new_len_react"=w396, "new_vol_react"=w393) -> ("Vr1"=w386:dbl, "Vr2"=w385:dbl, "Vr3"=w384:dbl, "Vr4"=w383:dbl, "Vr5"=w382:dbl)  [unwired: 1 in, 1 out]
                        n178 = local write "Vr1"(w386) -> ()
                        n179 = local write "Vr2"(w385) -> ()
                        n180 = local write "Vr3"(w384) -> ()
                        n181 = local write "Vr4"(w383) -> ()
                        n182 = local write "Vr5"(w382) -> ()
                      }
                      frame #4 {
                        n183 = local read "Setup Error"() -> (w416:bool)
                        n184 = case shown="True" w416 {
                          tunnel: [TRUE FALSE] -> w414
                          tunnel: ["" "Sytem setup has not been confirmed!"] -> w415
                          frame False {
                          }
                          frame True {
                            n185 = local read "Error Message"() -> (w421:string)
                            n186 = One Button Dialog(message=w421) -> ()  [unwired: 1 in, 1 out]
                          }
                        }
                        n187 = local write "System Confirm Not Clicked"(w415) -> ()
                        n188 = local write "Setup Confirm"(w414) -> ()
                      }
                    }
                  }
                }
              }
            }
            n189 = local read "Stop"() -> (w200:bool)
            n190 = Or(x=w201, y=w200) -> (x .or. y?=w199:bool)
            n191 = disable-structure shown="Disabled" {
              disable-tunnel: 400 -> [w207 _]
              frame Disabled {
                n192 = event shown="[1]" {
                  selector: _ -> [_ _]
                  dyn-events: _ -> [_ _]
                  timeout: w207 -> [_ _]
                  event Timeout {
                    n193 = event-data() -> ()  [unwired: 1 in, 3 out]
                  }
                  event #1 (no event record) {
                    n194 = event-data() -> ()  [unwired: 1 in, 6 out]
                    n195 = local read "Setup Confirm"() -> (w208:bool)
                    n196 = local read "Reaction Scheme Confirm"() -> (w209:bool)
                    n197 = Not(x=w208) -> (.not. x?=w211:bool)
                    n198 = And(x=w209, y=w211) -> (x .and. y?=w210:bool)
                    n199 = case shown="True" w210 {
                      frame False {
                      }
                      frame True {
                        w213 = u16 0 items=["                     Bypass", "                Hot Reactor", "                 Separator"] ("BAY 5")
                        w214 = u16 0 items=["                     Bypass", "                Hot Reactor", "                  Separator"] ("BAY 4")
                        w215 = u16 0 items=["                     Bypass", "                 Hot Reactor", "                  Separator"] ("BAY 3")
                        w216 = u16 0 items=["                     Bypass", "                Hot Reactor", "                  Separator"] ("BAY 2")
                        w217 = u16 0 items=["                 Bypass", "             Hot Reactor", "               Separator"] ("BAY 1")
                        n200 = local write "BAY 3"(w215) -> ()
                        n201 = local write "BAY 4"(w214) -> ()
                        n202 = local write "BAY 5"(w213) -> ()
                        n203 = local write "BAY 2"(w216) -> ()
                        n204 = local write "BAY 1"(w217) -> ()
                        n205 = local write "Synthesis Route Array"(string[][] [["3-Br-Pyridine _ Biphenyl", "K2CO3", "PhB(OH)2", "", "", ""]] ("Synthesis Route Array")) -> ()
                      }
                    }
                  }
                }
              }
              frame Enabled {
              }
            }
            n206 = disable-structure shown="Disabled" {
              disable-tunnel: 400 -> [w203 _]
              frame Disabled {
                n207 = event shown="[1]" {
                  selector: _ -> [_ _]
                  dyn-events: _ -> [_ _]
                  timeout: w203 -> [_ _]
                  event Timeout {
                    n208 = event-data() -> ()  [unwired: 1 in, 3 out]
                  }
                  event #1 (no event record) {
                    n209 = event-data() -> ()  [unwired: 1 in, 6 out]
                    n210 = call "File Dialog"("prompt"="Load previously saved xml file") -> ("selected path"=w205:path)  [unwired: 11 in, 3 out]
                    n211 = Path To String(path=w205) -> (string=w204:string)
                    n212 = script code="xmlDoc = xmlread(file_path);\nroot = xmlDoc.getDocumentElement();\nb = root.getChildNodes;\nrecipe = b.getElementsByTagName('Bay1').item(0);"("file_path"=w204) -> ()  [unwired: 1 in, 1 out]
                  }
                }
              }
              frame Enabled {
              }
            }
          }
        }
        frame #1 {
          n213 = local read "Stop"() -> (w423:bool)
          n214 = Not(x=w423) -> (.not. x?=w422:bool)
          n215 = case shown="True" w422 {
            tunnel: w424 -> [_ w427]
            frame False {
              "stop_button clicked" <- TRUE ("stop_button clicked")
            }
            frame True {
              # "Parameters Initilization"
              n216 = flat-sequence {
                tunnel: w427 -> [w429]
                tunnel: [w428] -> w426
                tunnel: w426 -> [w584]
                frame #0 {
                  # "Setup bays(RFID - verify)"
                  n217 = disable-structure shown="Disabled" {
                    frame Disabled {
                      n218 = local read "BAY 1"() -> ()  [unwired: 1 out]
                      n219 = local read "BAY 2"() -> ()  [unwired: 1 out]
                      n220 = local read "BAY 3"() -> ()  [unwired: 1 out]
                      n221 = local read "BAY 4"() -> ()  [unwired: 1 out]
                      n222 = local read "BAY 5"() -> ()  [unwired: 1 out]
                    }
                    frame Enabled {
                    }
                  }
                }
                frame #1 {
                  n223 = while {
                    tunnel: w429 -> [w432]
                    tunnel: [w431] -> w428
                    stop <- w435 stop-if-true
                    n224 = flat-sequence {
                      tunnel: [w445] -> w431
                      tunnel: w432 -> [w526]
                      tunnel: [w444] -> w430
                      frame #0 {
                        n225 = while {
                          stop <- w439 stop-if-true
                          n226 = event shown="[1] \"System Parameters Confirm Button\": Value Change" {
                            selector: _ -> [_ _]
                            dyn-events: _ -> [_ _]
                            timeout: u32 200 ("milliseconds to wait") -> [_ _]
                            tunnel: [FALSE TRUE] -> w437
                            event Timeout {
                              n227 = event-data() -> ()  [unwired: 1 in, 3 out]
                            }
                            event "System Parameters Confirm Button": Value Change {
                              n228 = event-data() -> ()  [unwired: 1 in, 5 out]
                              n229 = local write "System Parameters Confirm Button"(FALSE) -> ()
                            }
                          }
                          n230 = Wait (ms)(milliseconds to wait=u32 500) -> ()  [unwired: 1 out]
                          n231 = local read "Stop"() -> (w440:bool)
                          n232 = Or(x=w440, y=w437) -> (x .or. y?=w439:bool)
                        }
                      }
                      frame #1 {
                        w465 = 0 ("disabled index (col)")
                        w477 = 1 ("disabled index (col)")
                        # "Do while parameters have not been correctly entered"
                        n233 = local read "Bay Parameters"() -> (w464:T2)
                        n234 = local read "Synthesis Route Array"() -> (w478:string[][])
                        n235 = local read "Total Number of Experiments"() -> (w497:dbl)
                        n236 = Unbundle By Name(w464) -> ("Continue from previous optimization?"=w525:bool)
                        n237 = Unbundle By Name(w464) -> ("Excel File Name"=w527:string)
                        n238 = Unbundle By Name(w464) -> ("Matlab File"=w523:string)
                        n239 = Unbundle By Name(w464) -> ("Bay 1.Run at set flowrate"=w569:bool)
                        n240 = Unbundle By Name(w464) -> ("Bay 1.Pump 1 Flowrate"=w575:dbl)
                        n241 = Unbundle By Name(w464) -> ("Bay 1.Pump 2 Flowrate"=w574:dbl)
                        n242 = Unbundle By Name(w464) -> ("Bay 2.Run at set flowrate"=w567:bool)
                        n243 = Unbundle By Name(w464) -> ("Bay 2.Pump 3 Flowrate"=w573:dbl)
                        n244 = Unbundle By Name(w464) -> ("Bay 3.Pump 4 Flowrate"=w572:dbl)
                        n245 = Unbundle By Name(w464) -> ("Bay 3.Run at set flowrate"=w566:bool)
                        n246 = Unbundle By Name(w464) -> ("Bay 4.Run at set flowrate"=w563:bool)
                        n247 = Unbundle By Name(w464) -> ("Bay 4.Pump 5 Flowrate"=w571:dbl)
                        n248 = Unbundle By Name(w464) -> ("Bay 5.Pump 6 Flowrate"=w570:dbl)
                        n249 = Unbundle By Name(w464) -> ("Bay 5.Run at set flowrate"=w562:bool)
                        n250 = Index Array(array=w478, index (row)=3, index (col)=w477) -> (element=w471:string)
                        n251 = Index Array(array=w478, index (row)=2, index (col)=w477) -> (element=w469:string)
                        n252 = Index Array(array=w478, index (row)=1, index (col)=w477) -> (element=w467:string)
                        n253 = Index Array(array=w478, index (row)=0, index (col)=w477) -> (element=w480:string)
                        n254 = Index Array(array=w478, index (row)=4, index (col)=w477) -> (element=w473:string)
                        n255 = Index Array(array=w478, index (row)=5, index (col)=w477) -> (element=w475:string)
                        n256 = Build Array(w480, w467, w469, w471, w473, w475) -> (w481:string[])
                        n257 = Index Array(array=w478, index (row)=0 ("index"), index (col)=w465) -> (element=w503:string)
                        n258 = for {
                          tunnel: w481 -> [w577] mode=indexing
                          tunnel: [w576] -> w466 mode=indexing
                          n259 = script code="ctemp1 = str2num(c_temp);"("c_temp"=w577) -> ("ctemp1"=w576:dbl)  [unwired: 1 in, 1 out]
                        }
                        n260 = Boolean To (0,1)(Boolean=w567) -> (0, 1=w522:i16)
                        n261 = Boolean To (0,1)(Boolean=w563) -> (0, 1=w564:i16)
                        n262 = Boolean To (0,1)(Boolean=w566) -> (0, 1=w565:i16)
                        n263 = Boolean To (0,1)(Boolean=w525) -> (0, 1=w524:i16)
                        n264 = Boolean To (0,1)(Boolean=w569) -> (0, 1=w568:i16)
                        n265 = Boolean To (0,1)(Boolean=w562) -> (0, 1=w561:i16)
                        n266 = Index Array(array=w478, index (row)=1 ("index"), index (col)=w465) -> (element=w498:string)
                        n267 = Index Array(array=w478, index (row)=2 ("index"), index (col)=w465) -> (element=w499:string)
                        n268 = Unbundle By Name(w464) -> ("Bay 1.optimize_temp"=w560:bool)
                        n269 = Unbundle By Name(w464) -> ("Bay 1.optimize_tau"=w558:bool)
                        n270 = Unbundle By Name(w464) -> ("Bay 2.optimize_temp"=w556:bool)
                        n271 = Unbundle By Name(w464) -> ("Bay 2.optimize_tau"=w554:bool)
                        n272 = Unbundle By Name(w464) -> ("Bay 3.optimize_temp"=w552:bool)
                        n273 = Unbundle By Name(w464) -> ("Bay 3.optimize_tau"=w550:bool)
                        n274 = Unbundle By Name(w464) -> ("Bay 4.optimize_temp"=w548:bool)
                        n275 = Unbundle By Name(w464) -> ("Bay 4.optimize_tau"=w546:bool)
                        n276 = Index Array(array=w478, index (row)=3 ("index"), index (col)=w465) -> (element=w500:string)
                        n277 = Boolean To (0,1)(Boolean=w548) -> (0, 1=w547:i16)
                        n278 = Boolean To (0,1)(Boolean=w546) -> (0, 1=w545:i16)
                        n279 = Index Array(array=w478, index (row)=4 ("index"), index (col)=w465) -> (element=w501:string)
                        n280 = Boolean To (0,1)(Boolean=w550) -> (0, 1=w549:i16)
                        n281 = Boolean To (0,1)(Boolean=w556) -> (0, 1=w555:i16)
                        n282 = Boolean To (0,1)(Boolean=w560) -> (0, 1=w559:i16)
                        n283 = Boolean To (0,1)(Boolean=w554) -> (0, 1=w553:i16)
                        n284 = Boolean To (0,1)(Boolean=w558) -> (0, 1=w557:i16)
                        n285 = Boolean To (0,1)(Boolean=w552) -> (0, 1=w551:i16)
                        n286 = Unbundle By Name(w464) -> ("Bay 5.optimize_temp"=w544:bool)
                        n287 = Unbundle By Name(w464) -> ("Bay 5.optimize_tau"=w542:bool)
                        n288 = Index Array(array=w478, index (row)=5 ("index"), index (col)=w465) -> (element=w502:string)
                        n289 = Boolean To (0,1)(Boolean=w544) -> (0, 1=w543:i16)
                        n290 = Boolean To (0,1)(Boolean=w542) -> (0, 1=w541:i16)
                        n291 = Build Array(w559, w557, w555, w553, w551, w549, w547, w545, w543, w541) -> (w540:i16[])
                        n292 = Unbundle By Name(w464) -> ("Bay 1.Temperature Params"=w537:dbl[])
                        n293 = Unbundle By Name(w464) -> ("Bay 2.Temperature Params"=w536:dbl[])
                        n294 = Unbundle By Name(w464) -> ("Bay 2.Resisdence time params"=w531:dbl[])
                        n295 = Unbundle By Name(w464) -> ("Bay 3.Temperature Params"=w535:dbl[])
                        n296 = Unbundle By Name(w464) -> ("Bay 3.Resisdence time params"=w530:dbl[])
                        n297 = Unbundle By Name(w464) -> ("Bay 4.Temperature Params"=w534:dbl[])
                        n298 = Unbundle By Name(w464) -> ("Bay 4.Resisdence time params"=w529:dbl[])
                        n299 = Unbundle By Name(w464) -> ("Bay 5.Temperature Params"=w533:dbl[])
                        n300 = Unbundle By Name(w464) -> ("Bay 5.Resisdence time params"=w528:dbl[])
                        n301 = Unbundle By Name(w464) -> ("Bay 1.pump params 2"=w496:dbl[])
                        n302 = Unbundle By Name(w464) -> ("Bay 1.pump params 1"=w532:dbl[])
                        n303 = Unbundle By Name(w464) -> ("Bay 1.Run at set temperature"=w487:bool)
                        n304 = Unbundle By Name(w464) -> ("Bay 2.Run at set temperature"=w485:bool)
                        n305 = Unbundle By Name(w464) -> ("Bay 3.Run at set temperature"=w484:bool)
                        n306 = Unbundle By Name(w464) -> ("Bay 4.Run at set temperature"=w483:bool)
                        n307 = Unbundle By Name(w464) -> ("Bay 5.Run at set temperature"=w482:bool)
                        n308 = Unbundle By Name(w464) -> ("Bay 3.Temperature"=w493:dbl)
                        n309 = Unbundle By Name(w464) -> ("Bay 1.Temperature"=w495:dbl)
                        n310 = Unbundle By Name(w464) -> ("Bay 2.Temperature"=w494:dbl)
                        n311 = Unbundle By Name(w464) -> ("Bay 4.Temperature"=w492:dbl)
                        n312 = Unbundle By Name(w464) -> ("Bay 5.Temperature"=w491:dbl)
                        n313 = Unbundle By Name(w464) -> ("Bay 3.pump_num_ratio"=w516:dbl)
                        n314 = Unbundle By Name(w464) -> ("Bay 4.pump_num_ratio"=w513:dbl)
                        n315 = Unbundle By Name(w464) -> ("Bay 5.pump_num_ratio"=w510:dbl)
                        n316 = Unbundle By Name(w464) -> ("Bay 2.pump_num_ratio"=w519:dbl)
                        n317 = Unbundle By Name(w464) -> ("Bay 4.pump_at_ratio"=w515:bool)
                        n318 = Boolean To (0,1)(Boolean=w515) -> (0, 1=w514:i16)
                        n319 = Unbundle By Name(w464) -> ("Bay 3.pump_at_ratio"=w518:bool)
                        n320 = Boolean To (0,1)(Boolean=w518) -> (0, 1=w517:i16)
                        n321 = Unbundle By Name(w464) -> ("Bay 5.pump_at_ratio"=w512:bool)
                        n322 = Boolean To (0,1)(Boolean=w512) -> (0, 1=w511:i16)
                        n323 = Unbundle By Name(w464) -> ("Bay 2.pump_at_ratio"=w521:bool)
                        n324 = Boolean To (0,1)(Boolean=w521) -> (0, 1=w520:i16)
                        n325 = Build Array(w495, w494, w493, w492, w491) -> (w490:dbl[])
                        n326 = Build Array(w487, w485, w484, w483, w482) -> (w486:bool[])
                        n327 = for {
                          N: 5 -> [_]
                          tunnel: w486 -> [w581] mode=indexing
                          tunnel: [w580] -> w488 mode=indexing
                          n328 = Select(t=1.0, s=w581, f=0.0) -> (s? t:f=w580:dbl)
                        }
                        n329 = Unbundle By Name(w464) -> ("Internal Standard?"=w455:bool)
                        n330 = Unbundle By Name(w464) -> ("increas_decrease_hplc_peak"=w456:bool)
                        n331 = Unbundle By Name(w464) -> ("Hplc Wait time(min)"=w448:dbl)
                        n332 = Unbundle By Name(w464) -> ("Total Number of Experiments 2"=w447:dbl)
                        n333 = Unbundle By Name(w464) -> ("hplc_start"=w452:dbl)
                        n334 = Unbundle By Name(w464) -> ("ISTD start"=w450:dbl)
                        n335 = Unbundle By Name(w464) -> ("hplc_end"=w451:dbl)
                        n336 = Unbundle By Name(w464) -> ("throughput_yield"=w457:bool)
                        n337 = Unbundle By Name(w464) -> ("ISTD end"=w449:dbl)
                        n338 = Select(t=1.0, s=w456, f=0.0) -> (s? t:f=w454:dbl)
                        n339 = Select(t=1.0, s=w455, f=0.0) -> (s? t:f=w453:dbl)
                        n340 = Select(t=0.0, s=w457, f=1.0) -> (s? t:f=w446:dbl)
                        n341 = script code="system_error = 0;\nnumPeaks = 1;\nstart_phase_time = 1;\nis_redo_exp = 0;\nFvalues = [];\nHPLC_Area = [];\n\nT1_span = [1 1]; T2_span = [1 1]; T3_span = [1 1]; T4_span = [1 1]; T5_span = [1 1];\nT_span = [T1_span;T2_span;T3_span;T4_span;T5_span];\n p1_span =  [1 1]; p2_span =  [1 1]; p3_span =  [1 1]; p4_span =  [1 1]; p5_span =  [1 1];  p6_span =  [1 1];\nOpt_params = [0 0 0 0 0 0 0 0 0 0 0];\nT_params = [T1_params;T2_params;T3_params;T4_params;T5_params];\npump_params = [pump1_params;pump2_params;pump3_params;pump4_params;pump5_params;pump6_params];\nopt_ctr = 0;ncall = 100;record_data = true;\nT1_SP = 23; T2_SP = 23; T3_SP = 23; T4_SP = 23; T5_SP = 23;\nT_span = [T1_span;T2_span;T3_span;T4_span;T5_span];\np_span = [p1_span;p2_span;p3_span;p4_span;p5_span;p6_span];\nno_errors = 1;\nP1 = 0; P2 =0; P3 = 0; P4 = 0; P5 = 0; P6 = 0;\nP = [P1, P2, P3,P4, P5, P6];\nis_first_set_of_exp = true;\nerror_message = 'System has no errors to report';\naddpath(genpath('C:\\Users\\HPLC\\Dropbox (MIT)\\MoD Files\\MATLAB'))\n%addpath(genpath('C:\\Users\\Admin\\Dropbox (MIT)\\MoD Files\\MATLAB'))\nallMSData = [];allHPLCData = [];allHPLCFile = [];\nBay_ratio = [0,Bay2_ratio,Bay3_ratio,Bay4_ratio,Bay5_ratio];\nBay_pump_ratio = [1, Bay2_pump_ratio, Bay3_pump_ratio, Bay4_pump_ratio, Bay5_pump_ratio];\nP_setrate = [P1_setrate, P2_setrate, P3_setrate, P4_setrate, P5_setrate, P6_setrate];\nuse_flowrate = [use_flowrate1, use_flowrate2,use_flowrate3, use_flowrate4, use_flowrate5];\npump_chem_name= []\nCurrExp = 1;\n% ****************************************************************************************************\n%Setup optimization\n   setup_optimization_params;\n   initialize_opt = 0;\n   nstop0 = 0;\n%*****************************************************************************************************\n% Setup excel and xml file writing\npath(path, pa);\nnumMSSig = 1;\nsetup_excel_output;\n%***************************************************************************************************\nredo = false;\nncall = ncall_in;"("use_flowrate1"=w568, "P1_setrate"=w575, "P2_setrate"=w574, "P3_setrate"=w573, "P4_setrate"=w572, "P5_setrate"=w571, "P6_setrate"=w570, "use_flowrate2"=w522, "use_flowrate3"=w565, "use_flowrate4"=w564, "use_flowrate5"=w561, "Optimize_params"=w540, "T1_params"=w537, "T2_params"=w536, "T3_params"=w535, "T4_params"=w534, "T5_params"=w533, "pump1_params"=w532, "pump3_params"=w531, "pump4_params"=w530, "pump5_params"=w529, "pump6_params"=w528, "xl_file"=w527, "pa"=w526, "Continue"=w524, "matlabsavefile"=w523, "Bay2_ratio"=w520, "Bay2_pump_ratio"=w519, "Bay3_ratio"=w517, "Bay3_pump_ratio"=w516, "Bay4_ratio"=w514, "Bay4_pump_ratio"=w513, "Bay5_ratio"=w511, "Bay5_pump_ratio"=w510, "pump1_chem"=w503, "pump6_chem"=w502, "pump5_chem"=w501, "pump4_chem"=w500, "pump3_chem"=w499, "pump2_chem"=w498, "Pump_concen"=w466, "ncall_in"=w497, "pump2_params"=w496, "T_SP"=w490, "Run_at_T_SP"=w488, "dcr_hplc_peak"=w454, "use_internal_std"=w453, "hplc_peak_start"=w452, "hplc_peak_end"=w451, "ISTD_start"=w450, "ISTD_end"=w449, "hplc_wait_time"=w448, "tot_num_exp"=w447, "throughput_yield"=w446) -> ("no_errors"=w539:dbl, "error_message"=w538:string)  [unwired: 1 in, 1 out]
                        n342 = Not Equal To 0?(x=w539) -> (x != 0?=w444:bool)
                        n343 = Not(x=w444) -> (.not. x?=w445:bool)
                        n344 = case shown="False" w445 {
                          tunnel: w538 -> [_ w583]
                          frame False {
                            n345 = local write "Setup Confirm 2"(TRUE ("Setup Confirm 2")) -> ()
                          }
                          frame True {
                            n346 = One Button Dialog(message=w583) -> ()  [unwired: 1 in, 1 out]
                          }
                        }
                      }
                    }
                    n347 = local read "Stop"() -> (w434:bool)
                    n348 = Or(x=w430, y=w434) -> (x .or. y?=w435:bool)
                    n349 = Wait (ms)(milliseconds to wait=u32 500) -> ()  [unwired: 1 out]
                  }
                }
                frame #2 {
                  n350 = local write "System Error"(w584) -> ()
                }
              }
            }
          }
        }
        frame #2 {
          # "Run Initial diagnostics"
        }
        frame #3 {
          # "Run System"
          n351 = while {
            tunnel: w585 -> [w1284]
            stop <- w1288 stop-if-true
            n352 = local read "running?"() -> (w1283:bool)
            n353 = local read "Temperature Control 1"() -> (w1285:bool)
            n354 = And(x=w1283, y=w1285) -> (x .and. y?=w1286:bool)
            n355 = case shown="True" w1286 {
              tunnel: w1284 -> [_ w1290]
              frame False {
                n356 = local write "Temp SS? 1"(TRUE ("Temp SS? 1")) -> ()
              }
              frame True {
                # "Bay 1 Temperature Controller"
                n357 = local read "Temperature SP 1"() -> (w1291:dbl)
                n358 = local read "Temperature 1"() -> (w1295:dbl)
                n359 = local read "SSR Duration 1"() -> (w1310:dbl)
                n360 = call-poly <vilib>:"PID Online Autotuning.vi"("setpoint"=w1291, "manipulated variable"=w1310, "autotuning parameters"=T9 {"type of controller"=enum."PID", "relay cycles"=3, "relay amplitude"=1.0, "control specifications"=enum."Normal", "PV noise level"=0.1} ("Autotuning Parameters R1"), "process variable"=w1295, "PID gains in"=T8 {"Proportional gain Kc"=0.38538, "Integral time Ti (sec)"=0.524375, "Derivative time Ti (sec)"=0.12585} ("PID gains 2")) -> ("setpoint out"=w1316:dbl, "process variable out"=w1315:dbl, "PID gains out"=w1312:T17)  [unwired: 6 in, 2 out]
                n361 = call <vilib>:"PID Autotuning (Temperature).vi"("desired temperature"=w1316, "measured temperature"=w1315, "plant parameters in"=w1312, "output range"=cluster{"output high":dbl, "output low":dbl} {"output high"=3.0, "output low"=-1.0} ("Output range")) -> ("output"=w1308:dbl)  [unwired: 12 in, 3 out]
                n362 = local write "SSR Duration 1"(w1308) -> ()
                n363 = Subtract(x=w1291, y=w1295) -> (x-y=w1302:dbl)
                n364 = Absolute Value(x=w1302) -> (abs(x)=w1305:dbl)
                n365 = Multiply(x=1000.0, y=w1308) -> (x*y=w1306:dbl)
                n366 = Greater Than 0?(x=w1306) -> (x > 0?=w1300:bool)
                n367 = Less Or Equal?(x=w1305, y=1.2) -> (x <= y?=w1303:bool)
                n368 = Greater?(x=w1291, y=w1295) -> (0:w1301:bool)
                n369 = And(x=w1300, y=w1301) -> (x .and. y?=w1298:bool)
                n370 = local write "Temp SS? 1"(w1303) -> ()
                n371 = Subtract(x=w1295, y=10.0) -> (x-y=w1296:dbl)
                n372 = Less?(x=w1296, y=w1291) -> (x < y?=w1299:bool)
                n373 = And(x=w1299, y=w1298) -> (x .and. y?=w1297:bool)
                n374 = case shown="True" w1297 {
                  tunnel: [errorcluster {"status"=FALSE, "code"=0, "source"=""} ("error out") w1326] -> _
                  tunnel: 2 -> [_ w1323]
                  tunnel: w1306 -> [w1320 w1324]
                  tunnel: [0.0 w1328] -> w1293
                  tunnel: w1291 -> [_ w1327]
                  tunnel: w1290 -> [_ w1325]
                  frame False {
                    n375 = Absolute Value(x=w1320) -> (abs(x)=w1321:dbl)
                    n376 = Wait (ms)(milliseconds to wait=w1321) -> ()  [unwired: 1 out]
                  }
                  frame True {
                    n377 = call "TurnOnRelayArduino.vi"("channel"=w1323, "duration"=w1324, "LINX Resource"=w1325) -> ("error out"=w1326:errorcluster)  [unwired: 7 in, 1 out]
                    n378 = script code="tempdiff1= SP1 - T1;\nif tempdiff1 > 10\n  if slope1 < .01\n     temp_check1 = temp_check1 + 1;\n  else\n      temp_check1 =0;\n  end\nend\n\nif temp_check1 > 9\n  temp_error1 = 1\nend"("SP1"=w1327) -> ("temp_error1"=w1328:dbl)  [unwired: 1 in, 1 out]
                  }
                }
                n379 = Not Equal To 0?(x=w1293) -> (x != 0?=w1292:bool)
                n380 = case shown="True" w1292 {
                  frame False {
                  }
                  frame True {
                    n381 = local write "Error Message"("Bay 1 Temperature Heating Error") -> ()
                  }
                }
                n382 = case shown="True" w1292 {
                  tunnel: w1292 -> [_ w1318]
                  frame False {
                  }
                  frame True {
                    n383 = local write "System Error"(w1318) -> ()
                    n384 = local write "Stop"(w1318) -> ()
                  }
                }
              }
            }
            n385 = Wait (ms)(milliseconds to wait=u32 400) -> ()  [unwired: 1 out]
            n386 = local read "Stop"() -> (w1288:bool)
          }
          n387 = local read "Bay Parameters"() -> (w589:T2)
          n388 = while {
            tunnel: w585 -> [w1238]
            stop <- w1242 stop-if-true
            n389 = local read "running?"() -> (w1237:bool)
            n390 = local read "Temperature Control 2"() -> (w1239:bool)
            n391 = And(x=w1237, y=w1239) -> (x .and. y?=w1240:bool)
            n392 = case shown="True" w1240 {
              tunnel: w1238 -> [_ w1244]
              frame False {
                n393 = local write "Temp SS? 2"(TRUE ("Temp SS? 2")) -> ()
              }
              frame True {
                # "Bay 2 Temperature Controller"
                n394 = local read "Temperature SP 2"() -> (w1246:dbl)
                n395 = local read "Temperature 2"() -> (w1249:dbl)
                n396 = local read "SSR Duration 2"() -> (w1267:dbl)
                n397 = call-poly <vilib>:"PID Online Autotuning.vi"("setpoint"=w1246, "manipulated variable"=w1267, "autotuning parameters"=T9 {"type of controller"=enum."PID", "relay cycles"=3, "relay amplitude"=1.0, "control specifications"=enum."Normal", "PV noise level"=0.1} ("Autotuning Parameters R1"), "process variable"=w1249, "PID gains in"=T8 {"Proportional gain Kc"=0.38538, "Integral time Ti (sec)"=0.524375, "Derivative time Ti (sec)"=0.12585} ("PID gains 2")) -> ("setpoint out"=w1265:dbl, "process variable out"=w1264:dbl, "PID gains out"=w1270:T17)  [unwired: 6 in, 2 out]
                n398 = call <vilib>:"PID Autotuning (Temperature).vi"("desired temperature"=w1265, "measured temperature"=w1264, "plant parameters in"=w1270, "output range"=cluster{"output high":dbl, "output low":dbl} {"output high"=3.0, "output low"=-1.0} ("Output range")) -> ("output"=w1260:dbl)  [unwired: 12 in, 3 out]
                n399 = local write "SSR Duration 2"(w1260) -> ()
                n400 = Greater?(x=w1246, y=w1249) -> (0:w1255:bool)
                n401 = Multiply(x=1000.0, y=w1260) -> (x*y=w1262:dbl)
                n402 = Greater Than 0?(x=w1262) -> (x > 0?=w1254:bool)
                n403 = And(x=w1254, y=w1255) -> (x .and. y?=w1252:bool)
                n404 = Subtract(x=w1246, y=w1249) -> (x-y=w1257:dbl)
                n405 = Absolute Value(x=w1257) -> (abs(x)=w1259:dbl)
                n406 = Subtract(x=w1249, y=10.0) -> (x-y=w1251:dbl)
                n407 = Less Or Equal?(x=w1259, y=1.2) -> (x <= y?=w1256:bool)
                n408 = local write "Temp SS? 2"(w1256) -> ()
                n409 = Less?(x=w1251, y=w1246) -> (x < y?=w1253:bool)
                n410 = And(x=w1253, y=w1252) -> (x .and. y?=w1248:bool)
                n411 = case shown="True" w1248 {
                  tunnel: [errorcluster {"status"=FALSE, "code"=0, "source"=""} ("error out") w1280] -> _
                  tunnel: 3 -> [_ w1277]
                  tunnel: w1262 -> [w1274 w1278]
                  tunnel: [0.0 w1282] -> w1247
                  tunnel: w1246 -> [_ w1281]
                  tunnel: w1244 -> [_ w1279]
                  frame False {
                    n412 = Absolute Value(x=w1274) -> (abs(x)=w1275:dbl)
                    n413 = Wait (ms)(milliseconds to wait=w1275) -> ()  [unwired: 1 out]
                  }
                  frame True {
                    n414 = call "TurnOnRelayArduino.vi"("channel"=w1277, "duration"=w1278, "LINX Resource"=w1279) -> ("error out"=w1280:errorcluster)  [unwired: 7 in, 1 out]
                    n415 = script code="tempdiff2= SP2 - T2;\nif tempdiff2 > 10\n  if slope2 < .01\n     temp_check2 = temp_check2 + 1;\n  else\n      temp_check2 =0;\n  end\nend\n\nif temp_check2 > 9\n  temp_error2 = 1\nend"("SP2"=w1281) -> ("temp_error2"=w1282:dbl)  [unwired: 1 in, 1 out]
                  }
                }
                n416 = Not Equal To 0?(x=w1247) -> (x != 0?=w1245:bool)
                n417 = case shown="True" w1245 {
                  frame False {
                  }
                  frame True {
                    n418 = local write "Error Message"("Bay 2 Temperature Heating Error") -> ()
                  }
                }
                n419 = case shown="True" w1245 {
                  tunnel: w1245 -> [_ w1272]
                  frame False {
                  }
                  frame True {
                    n420 = local write "Stop"(w1272) -> ()
                    n421 = local write "System Error"(w1272) -> ()
                  }
                }
              }
            }
            n422 = local read "Stop"() -> (w1242:bool)
            n423 = Wait (ms)(milliseconds to wait=u32 400) -> ()  [unwired: 1 out]
          }
          n424 = local read "Stop"() -> (w586:bool)
          n425 = Not(x=w586) -> (.not. x?=w588:bool)
          n426 = case shown="True" w588 {
            tunnel: w589 -> [_ w594]
            tunnel: w587 -> [_ w593]
            tunnel: w585 -> [_ w592]
            frame False {
            }
            frame True {
              n427 = while {
                tunnel: w594 -> [w608]
                tunnel: w593 -> [w600]
                tunnel: w592 -> [w595]
                i -> [w607]
                stop <- w601 stop-if-true
                n428 = local read "running?"() -> (w596:bool)
                n429 = Wait (ms)(milliseconds to wait=u32 1000) -> ()  [unwired: 1 out]
                n430 = Increment(x=w607) -> (x+1=w597:i32)
                n431 = case shown="True" w596 {
                  tunnel: w607 -> [w613 _]
                  tunnel: w608 -> [_ _]
                  tunnel: [w615 w619] -> w598
                  tunnel: [0.0 w620] -> w603
                  tunnel: w600 -> [_ w618]
                  tunnel: w595 -> [_ w616]
                  frame False {
                    # "STANDBY MODE"
                    n432 = Add(x=w613, y=2.0) -> (x+y=w615:dbl)
                  }
                  frame True {
                    n433 = flat-sequence {
                      tunnel: w618 -> [w622]
                      tunnel: [w622] -> w617
                      tunnel: [w631] -> w620
                      tunnel: [200.0] -> w619
                      tunnel: w617 -> [w629]
                      tunnel: w616 -> [w623]
                      frame #0 {
                        n434 = local write "stop_xl_write"(FALSE ("stop_xl_write")) -> ()
                      }
                      frame #1 {
                        # "Increase flowrate of dilution stream"
                        # "Wait mixed stream reaches SL"
                        # "SNOBFIT"
                        # "Optimize"
                        # "Run Experimental Conditions"
                        # "Optimize/Synthesize"
                        n435 = local read "Stop"() -> (w626:bool)
                        n436 = Not(x=w626) -> (.not. x?=w625:bool)
                        n437 = case shown="True" w625 {
                          tunnel: [1.0 w650] -> w634
                          tunnel: [w642 w649] -> w628
                          tunnel: [0.0 w648] -> w627
                          tunnel: [w642 w647] -> w624
                          frame False {
                            w642 = dbl[] []
                          }
                          frame True {
                            n438 = script code="optimization_main_loop"() -> ("Conditions_Array"=w649:dbl[], "opt_ctr"=w650:dbl, "P_tot"=w648:dbl, "tau_array"=w647:dbl[], "experiment_history"=w645:dbl[][])  [unwired: 1 in, 1 out]
                            n439 = call-poly <vilib>:"Array To Matrix.vi"("Real 2D Array"=w645) -> ("Real Matrix"=w646:T18)
                            n440 = local write "experiment history"(w646) -> ()
                          }
                        }
                        "P_tot" <- w627
                        n441 = local read "COMM Port :: Milligat Pumps"() -> (w635:refnum<visa-resource-name>)
                        n442 = Equal?(x=w634, y=1.0) -> (x = y?=w632:bool)
                        n443 = flat-sequence {
                          tunnel: w628 -> [w1082]
                          tunnel: w624 -> [w1076]
                          frame #0 {
                            # "Start recording data"
                            n444 = Index Array(array=w1082, index=5) -> (element=w1094:dbl)
                            n445 = Index Array(array=w1082, index=0) -> (element=w1089:dbl)
                            n446 = Index Array(array=w1082, index=1) -> (element=w1090:dbl)
                            n447 = Index Array(array=w1082, index=2) -> (element=w1092:dbl)
                            n448 = Index Array(array=w1082, index=3) -> (element=w1091:dbl)
                            n449 = Index Array(array=w1082, index=4) -> (element=w1093:dbl)
                            n450 = local write "Pump setpoint(ul/min) 2"(w1090) -> ()
                            n451 = local write "Pump setpoint(ul/min) 4"(w1092) -> ()
                            n452 = local write "Pump setpoint(ul/min) 5"(w1093) -> ()
                            n453 = local write "Pump setpoint(ul/min) 3"(w1091) -> ()
                            n454 = local write "Pump setpoint(ul/min) 6"(w1094) -> ()
                            n455 = local write "Pump setpoint(ul/min) 1"(w1089) -> ()
                            n456 = Index Array(array=w1076, index=0) -> (element=w1081:dbl)
                            n457 = Index Array(array=w1076, index=4) -> (element=w1080:dbl)
                            n458 = Index Array(array=w1076, index=3) -> (element=w1079:dbl)
                            n459 = Index Array(array=w1076, index=2) -> (element=w1078:dbl)
                            n460 = Index Array(array=w1076, index=1) -> (element=w1077:dbl)
                            n461 = local write "tau 2"(w1077) -> ()
                            n462 = local write "tau 3"(w1078) -> ()
                            n463 = local write "tau 4"(w1079) -> ()
                            n464 = local write "tau 5"(w1080) -> ()
                            n465 = local write "tau 1"(w1081) -> ()
                          }
                        }
                        n466 = flat-sequence {
                          tunnel: w635 -> [w654]
                          tunnel: w628 -> [w653]
                          tunnel: w632 -> [w652]
                          tunnel: [w652] -> w641
                          tunnel: w629 -> [w651]
                          tunnel: w641 -> [w798]
                          tunnel: [w798] -> w640
                          tunnel: w640 -> [w818]
                          tunnel: [w816] -> w639
                          tunnel: w628 -> [w842]
                          tunnel: w639 -> [w841]
                          tunnel: w623 -> [w840]
                          tunnel: [w1012] -> w638
                          tunnel: w638 -> [w1025]
                          tunnel: [w1025] -> w637
                          tunnel: w637 -> [w1033]
                          tunnel: [w1033] -> w636
                          tunnel: [w1070] -> w631
                          tunnel: w636 -> [w1070]
                          frame #0 {
                            # "Setup pump flowrates and temperature setpoints"
                            n467 = stacked-sequence {
                              tunnel: w654 -> [w676 _ _ _ _]
                              tunnel: w654 -> [_ w716 _ _ _]
                              tunnel: w654 -> [_ _ w740 _ _]
                              tunnel: w654 -> [_ _ _ w764 _]
                              tunnel: w654 -> [_ _ _ _ w788]
                              tunnel: w653 -> [w673 w714 w738 w762 w785]
                              tunnel: w652 -> [w663 w707 w731 w755 w779]
                              tunnel: w651 -> [w661 _ _ _ _]
                              frame #0 {
                                # "Bay 1"
                                n468 = local read "Syringe_pump?"() -> (w662:bool)
                                n469 = Index Array(array=w673, index=0) -> (element=w671:dbl)
                                n470 = local read "BAY 1"() -> (w656:u16)
                                n471 = Index Array(array=w673, index=1) -> (element=w670:dbl)
                                n472 = Index Array(array=w673, index=6) -> (element=w669:dbl)
                                n473 = script code="MATLAB script"("P1"=w671, "P2"=w670, "T1_SP"=w669) -> ()  [unwired: 1 in, 1 out]
                                n474 = Less Or Equal?(x=w656, y=u16 4) -> (x <= y?=w658:bool)
                                n475 = Greater Or Equal?(x=w656, y=u16 1) -> (x >= y?=w659:bool)
                                n476 = And(x=w659, y=w658) -> (x .and. y?=w660:bool)
                                n477 = Greater Than 0?(x=w671) -> (x > 0?=w668:bool)
                                n478 = And(x=w668, y=w663) -> (x .and. y?=w667:bool)
                                n479 = Greater Than 0?(x=w670) -> (x > 0?=w666:bool)
                                n480 = And(x=w666, y=w663) -> (x .and. y?=w665:bool)
                                n481 = And(x=w660, y=w663) -> (x .and. y?=w664:bool)
                                n482 = case shown="False" w662 {
                                tunnel: w676 -> [w679 _]
                                tunnel: w670 -> [w678 w684]
                                tunnel: w665 -> [w677 w685]
                                tunnel: w661 -> [_ w683]
                                frame False {
                                n483 = case shown="False" w677 {
                                tunnel: w679 -> [w681 _]
                                tunnel: w678 -> [w680 _]
                                frame False {
                                n484 = call "PumpDispense.vi"("Flowrate(ul/min)"=w680, "Pump Address"="j", "Pump COMM Port"=w681) -> ()  [unwired: 7 in, 2 out]
                                }
                                frame True {
                                }
                                }
                                }
                                frame True {
                                n485 = case shown="False" w685 {
                                tunnel: w684 -> [_ w687]
                                tunnel: w683 -> [w686 w688]
                                frame False {
                                n486 = call <instrlib>:"Stop Pump.vi"("VISA resource name"=w686) -> ()  [unwired: 9 in, 2 out]
                                }
                                frame True {
                                w689 = u16 0 items=["Infuse", "Withdraw"] ("Run Direction (0:Infuse)")
                                w690 = u32 4 items=["milliliters per hour (ml/hr)", "milliliters per minute (ml/min)", "milliliters per second (ml/sec)", "microliters per hour (ul/hr)", "microliters per minute (ul/min)", "microliters per second (ul/sec)", "nanoliters per hour (nl/hr)", "nanoliters per minute (nl/min)", "nanoliters per second (nl/sec)", "picoliters per hour (pl/hr)", "picoliters per minute (pl/min)", "picoliters per second (pl/sec)"] ("Flow Rate Units (1:ml/min)")
                                w691 = u16 0 items=["Infuse", "Withdraw"] ("Pump Direction (0:Infuse)")
                                n487 = call <instrlib>:"Configure Flow Rate & Direction.vi"("VISA resource name"=w688, "Pump Direction (0:Infuse)"=w691, "Flow Rate (5.00)"=w687, "Flow Rate Units (1:ml/min)"=w690) -> ("VISA resource name out"=w692:refnum<visa-resource-name>)  [unwired: 10 in, 1 out]
                                n488 = call <instrlib>:"Start Pump.vi"("Run Direction (0:Infuse)"=w689, "VISA resource name"=w692) -> ()  [unwired: 8 in, 2 out]
                                }
                                }
                                }
                                }
                                n489 = case shown="False" w667 {
                                tunnel: w676 -> [w696 w698]
                                tunnel: w671 -> [_ w699]
                                frame False {
                                n490 = call "PumpStop.vi"("Pump Address"="g", "Pump COMM Port"=w696) -> ()  [unwired: 9 in, 1 out]
                                }
                                frame True {
                                n491 = call "PumpDispense.vi"("Flowrate(ul/min)"=w699, "Pump Address"="g", "Pump COMM Port"=w698) -> ()  [unwired: 7 in, 2 out]
                                }
                                }
                                n492 = case shown="True" w664 {
                                tunnel: w669 -> [_ w695]
                                frame False {
                                n493 = local write "Temperature Control 1"(FALSE) -> ()
                                }
                                frame True {
                                n494 = local write "Temperature SP 1"(w695) -> ()
                                n495 = local write "Temperature Control 1"(TRUE ("Temperature Control 1")) -> ()
                                }
                                }
                              }
                              frame #1 {
                                # "Bay 2"
                                n496 = local read "BAY 2"() -> (w703:u16)
                                n497 = Index Array(array=w714, index=2) -> (element=w711:dbl)
                                n498 = Index Array(array=w714, index=7) -> (element=w712:dbl)
                                n499 = script code="MATLAB script"("T2_SP"=w712, "P3"=w711) -> ()  [unwired: 1 in, 1 out]
                                n500 = Greater Than 0?(x=w711) -> (x > 0?=w709:bool)
                                n501 = And(x=w709, y=w707) -> (x .and. y?=w708:bool)
                                n502 = Greater Or Equal?(x=w703, y=u16 1) -> (x >= y?=w701:bool)
                                n503 = Less Or Equal?(x=w703, y=u16 4) -> (x <= y?=w706:bool)
                                n504 = And(x=w701, y=w706) -> (x .and. y?=w705:bool)
                                n505 = And(x=w705, y=w707) -> (x .and. y?=w710:bool)
                                n506 = case shown="True" w710 {
                                tunnel: w712 -> [_ w723]
                                frame False {
                                n507 = local write "Temperature Control 2"(FALSE) -> ()
                                }
                                frame True {
                                n508 = local write "Temperature Control 2"(TRUE ("Temperature Control 2")) -> ()
                                n509 = local write "Temperature SP 2"(w723) -> ()
                                }
                                }
                                n510 = case shown="False" w708 {
                                tunnel: w711 -> [_ w719]
                                tunnel: w716 -> [w717 w720]
                                frame False {
                                n511 = call "PumpStop.vi"("Pump Address"="i", "Pump COMM Port"=w717) -> ()  [unwired: 9 in, 1 out]
                                }
                                frame True {
                                n512 = call "PumpDispense.vi"("Flowrate(ul/min)"=w719, "Pump Address"="i", "Pump COMM Port"=w720) -> ()  [unwired: 7 in, 2 out]
                                }
                                }
                              }
                              frame #2 {
                                # "Bay 3"
                                n513 = local read "BAY 3"() -> (w726:u16)
                                n514 = Index Array(array=w738, index=3) -> (element=w735:dbl)
                                n515 = Not Equal To 0?(x=w735) -> (x != 0?=w734:bool)
                                n516 = Index Array(array=w738, index=8) -> (element=w736:dbl)
                                n517 = script code="MATLAB script"("T3_SP"=w736, "P4"=w735) -> ()  [unwired: 1 in, 1 out]
                                n518 = Less Or Equal?(x=w726, y=u16 4) -> (x <= y?=w730:bool)
                                n519 = Greater Or Equal?(x=w726, y=u16 1) -> (x >= y?=w727:bool)
                                n520 = And(x=w727, y=w730) -> (x .and. y?=w725:bool)
                                n521 = And(x=w725, y=w731) -> (x .and. y?=w732:bool)
                                n522 = And(x=w734, y=w731) -> (x .and. y?=w733:bool)
                                n523 = case shown="True" w733 {
                                tunnel: w735 -> [_ w743]
                                tunnel: w740 -> [w741 w744]
                                frame False {
                                n524 = call "PumpStop.vi"("Pump Address"="e", "Pump COMM Port"=w741) -> ()  [unwired: 9 in, 1 out]
                                }
                                frame True {
                                n525 = call "PumpDispense.vi"("Flowrate(ul/min)"=w743, "Pump Address"="e", "Pump COMM Port"=w744) -> ()  [unwired: 7 in, 2 out]
                                }
                                }
                                n526 = case shown="False" w732 {
                                tunnel: w736 -> [_ w747]
                                frame False {
                                n527 = local write "Temperature Control 3"(FALSE) -> ()
                                }
                                frame True {
                                n528 = local write "Temperature Control 3"(TRUE ("Temperature Control 3")) -> ()
                                n529 = local write "Temperature SP 3"(w747) -> ()
                                }
                                }
                              }
                              frame #3 {
                                # "Bay 4"
                                n530 = Index Array(array=w762, index=9) -> (element=w759:dbl)
                                n531 = Index Array(array=w762, index=4) -> (element=w760:dbl)
                                n532 = script code="MATLAB script"("P5"=w760, "T4_SP"=w759) -> ()  [unwired: 1 in, 1 out]
                                n533 = Not Equal To 0?(x=w760) -> (x != 0?=w758:bool)
                                n534 = local read "BAY 4"() -> (w749:u16)
                                n535 = And(x=w758, y=w755) -> (x .and. y?=w757:bool)
                                n536 = Less Or Equal?(x=w749, y=u16 4) -> (x <= y?=w754:bool)
                                n537 = Greater Or Equal?(x=w749, y=u16 1) -> (x >= y?=w751:bool)
                                n538 = And(x=w751, y=w754) -> (x .and. y?=w750:bool)
                                n539 = And(x=w750, y=w755) -> (x .and. y?=w756:bool)
                                n540 = case shown="False" w757 {
                                tunnel: w764 -> [w765 w768]
                                tunnel: w760 -> [_ w767]
                                frame False {
                                n541 = call "PumpStop.vi"("Pump Address"="f", "Pump COMM Port"=w765) -> ()  [unwired: 9 in, 1 out]
                                }
                                frame True {
                                n542 = call "PumpDispense.vi"("Flowrate(ul/min)"=w767, "Pump Address"="f", "Pump COMM Port"=w768) -> ()  [unwired: 7 in, 2 out]
                                }
                                }
                                n543 = case shown="True" w756 {
                                tunnel: w759 -> [_ w771]
                                frame False {
                                n544 = local write "Temperature Control 4"(FALSE ("Temperature Control 4")) -> ()
                                }
                                frame True {
                                n545 = local write "Temperature SP 4"(w771) -> ()
                                n546 = local write "Temperature Control 4"(TRUE ("Temperature Control 5")) -> ()
                                }
                                }
                              }
                              frame #4 {
                                # "Bay 5"
                                n547 = Index Array(array=w785, index=5) -> (element=w783:dbl)
                                n548 = Index Array(array=w785, index=4) -> (element=w784:dbl)
                                n549 = script code="MATLAB script"("T5_SP"=w784, "P6"=w783) -> ()  [unwired: 1 in, 1 out]
                                n550 = Not Equal To 0?(x=w783) -> (x != 0?=w781:bool)
                                n551 = And(x=w781, y=w779) -> (x .and. y?=w780:bool)
                                n552 = local read "BAY 5"() -> (w774:u16)
                                n553 = Less Or Equal?(x=w774, y=u16 4) -> (x <= y?=w778:bool)
                                n554 = Greater Or Equal?(x=w774, y=u16 1) -> (x >= y?=w775:bool)
                                n555 = case shown="False" w780 {
                                tunnel: w788 -> [w789 w792]
                                tunnel: w783 -> [_ w791]
                                frame False {
                                n556 = call "PumpStop.vi"("Pump Address"="h", "Pump COMM Port"=w789) -> ()  [unwired: 9 in, 1 out]
                                }
                                frame True {
                                n557 = call "PumpDispense.vi"("Flowrate(ul/min)"=w791, "Pump Address"="h", "Pump COMM Port"=w792) -> ()  [unwired: 7 in, 2 out]
                                }
                                }
                                n558 = And(x=w775, y=w778) -> (x .and. y?=w773:bool)
                                n559 = And(x=w773, y=w779) -> (x .and. y?=w782:bool)
                                n560 = case shown="True" w782 {
                                tunnel: w784 -> [_ w795]
                                frame False {
                                n561 = local write "Temperature Control 5"(FALSE ("Temperature Control 5")) -> ()
                                }
                                frame True {
                                n562 = local write "Temperature SP 5"(w795) -> ()
                                n563 = local write "Temperature Control 5"(TRUE ("Temperature Control 5")) -> ()
                                }
                                }
                              }
                            }
                          }
                          frame #1 {
                            # "Wait till Steady State temperature readings on all bays"
                            n564 = while {
                              tunnel: w798 -> [w799]
                              stop <- w800 stop-if-true
                              n565 = flat-sequence {
                                tunnel: [w803] -> w800
                                tunnel: w799 -> [w802]
                                frame #0 {
                                n566 = Wait (ms)(milliseconds to wait=u32 1500) -> ()  [unwired: 1 out]
                                }
                                frame #1 {
                                n567 = local read "Temp SS? 2"() -> (w806:bool)
                                n568 = local read "Temp SS? 3"() -> (w807:bool)
                                n569 = local read "Temp SS? 4"() -> (w808:bool)
                                n570 = local read "Temp SS? 5"() -> (w809:bool)
                                n571 = local read "Temp SS? 1"() -> (w805:bool)
                                n572 = Not(x=w802) -> (.not. x?=w815:bool)
                                n573 = local read "Stop"() -> (w804:bool)
                                n574 = And(x=w807, y=w808) -> (x .and. y?=w811:bool)
                                n575 = And(x=w805, y=w806) -> (x .and. y?=w812:bool)
                                n576 = And(x=w812, y=w811) -> (x .and. y?=w810:bool)
                                n577 = And(x=w810, y=w809) -> (x .and. y?=w813:bool)
                                n578 = Or(x=w815, y=w813) -> (x .or. y?=w814:bool)
                                n579 = Or(x=w814, y=w804) -> (x .or. y?=w803:bool)
                                }
                              }
                            }
                            n580 = local write "Calculate condition"(TRUE ("Calculate condition")) -> ()
                          }
                          frame #2 {
                            n581 = flat-sequence {
                              tunnel: w818 -> [w820]
                              tunnel: [w820] -> w817
                              tunnel: w817 -> [w827]
                              tunnel: [w827] -> w816
                              frame #0 {
                                n582 = local write "Equlibrating Temperature"(TRUE) -> ()
                              }
                              frame #1 {
                                # "Wait 1.5 system volumes"
                                n583 = local read "Number of System Flushes per condtion"() -> (w824:dbl)
                                n584 = local read "Extra system dead volume"() -> (w825:dbl)
                                n585 = script code="start = tic;\nP_tot = P1+P2+P3+P4+P5+P6;\nif P_tot >0\n  extra_res = extr_sys_dead_vol/P_tot;\nelse\n   extra_res =0;\nend\ntotal_sys_res = tau1 + tau2 + tau3 + tau4 + tau5 + extra_res;\ntotal_wait_time = total_sys_res*num_flush_per_cond*60;"("extr_sys_dead_vol"=w825, "num_flush_per_cond"=w824) -> ("??"=w828:errorcluster, "total_wait_time"=w822:dbl, "total_sys_res"=→"Total System Resisdence Time(min)":dbl)  [unwired: 1 in]
                                n586 = Divide(x=w822, y=60.0) -> (x/y=→"total_flush_time":dbl)
                                n587 = while {
                                tunnel: w827 -> [w830]
                                tunnel: w828 -> [w833]
                                stop <- w834 stop-if-true
                                # "Check if system is flushed every 10 seconds"
                                n588 = script code="end1 = toc(start);\nflush_time = 0;\nif end1 > total_wait_time\n   flush_time = 1;\nend\ncurr_wait_time = end1 /60;"("??"=w833) -> ("flush_time"=w837:dbl, "curr_wait_time"=w832:dbl)  [unwired: 1 out]
                                "curr_wait_time" <- w832
                                n589 = Not Equal To 0?(x=w837) -> (x != 0?=w836:bool)
                                n590 = Multiply(x=60.0, y=w832) -> ()  [unwired: 1 out]
                                n591 = local read "Stop"() -> (w839:bool)
                                n592 = Or(x=w836, y=w839) -> (x .or. y?=w835:bool)
                                n593 = Not(x=w830) -> (.not. x?=w829:bool)
                                n594 = Wait (ms)(milliseconds to wait=u32 10000) -> ()  [unwired: 1 out]
                                n595 = Or(x=w835, y=w829) -> (x .or. y?=w834:bool)
                                }
                              }
                            }
                          }
                          frame #3 {
                            # "Collect HPLC Data"
                            n596 = flat-sequence {
                              tunnel: w842 -> [w851]
                              tunnel: w841 -> [w850]
                              tunnel: w840 -> [w849]
                              tunnel: w840 -> [w848]
                              frame #0 {
                                n597 = local read "pause for ms"() -> (w845:bool)
                                n598 = case shown="True" w845 {
                                frame False {
                                }
                                frame True {
                                n599 = One Button Dialog(message="Press OK to Analyze Data", button name ("OK")="OK" ("Left Button Text (\"Yes\")")) -> ()  [unwired: 1 out]
                                }
                                }
                                n600 = local write "Flushing System"(TRUE ("Flushing System")) -> ()
                                "System Flushed?" <- TRUE ("System Flushed?")
                              }
                              frame #1 {
                                n601 = flat-sequence {
                                tunnel: w851 -> [w856]
                                tunnel: w850 -> [_]
                                tunnel: w849 -> [w855]
                                tunnel: w848 -> [w854]
                                frame #0 {
                                }
                                frame #1 {
                                n602 = flat-sequence {
                                tunnel: w856 -> [w857]
                                tunnel: w855 -> [w929]
                                tunnel: w856 -> [_]
                                tunnel: [w949] -> w853
                                tunnel: [w948] -> w852
                                tunnel: w854 -> [w947]
                                tunnel: w853 -> [w982]
                                tunnel: w852 -> [w981]
                                frame #0 {
                                n603 = local read "COMM Port :: Milligat Pumps"() -> (w859:refnum<visa-resource-name>)
                                n604 = stacked-sequence {
                                tunnel: w859 -> [w862 w874 w892 w897 w906 w919]
                                tunnel: w857 -> [w861 w870 w889 w899 w908 w915]
                                tunnel: 1.0 ("Flowrate(ul/min)") -> [w860 w869 w887 w896 w905 w914]
                                frame #0 {
                                n605 = Index Array(array=w861, index=0) -> (element=w864:dbl)
                                n606 = Greater Than 0?(x=w864) -> (x > 0?=w863:bool)
                                n607 = case shown="True" w863 {
                                tunnel: w862 -> [_ w867]
                                tunnel: w860 -> [_ w866]
                                frame False {
                                }
                                frame True {
                                n608 = call "PumpDispense.vi"("Flowrate(ul/min)"=w866, "Pump Address"="g", "Pump COMM Port"=w867) -> ()  [unwired: 7 in, 2 out]
                                }
                                }
                                }
                                frame #1 {
                                n609 = Index Array(array=w870, index=1) -> (element=w872:dbl)
                                n610 = Greater Than 0?(x=w872) -> (x > 0?=w871:bool)
                                n611 = case shown="False" w871 {
                                tunnel: w869 -> [_ w876]
                                tunnel: w874 -> [_ w875]
                                frame False {
                                }
                                frame True {
                                n612 = local read "Syringe_pump?"() -> (w877:bool)
                                n613 = case shown="False" w877 {
                                tunnel: w876 -> [w878 _]
                                tunnel: w875 -> [w879 _]
                                frame False {
                                n614 = call "PumpDispense.vi"("Flowrate(ul/min)"=w878, "Pump Address"="j", "Pump COMM Port"=w879) -> ()  [unwired: 7 in, 2 out]
                                }
                                frame True {
                                w886 = u16 0 items=["Infuse", "Withdraw"] ("Run Direction (0:Infuse)")
                                w882 = u32 4 items=["milliliters per hour (ml/hr)", "milliliters per minute (ml/min)", "milliliters per second (ml/sec)", "microliters per hour (ul/hr)", "microliters per minute (ul/min)", "microliters per second (ul/sec)", "nanoliters per hour (nl/hr)", "nanoliters per minute (nl/min)", "nanoliters per second (nl/sec)", "picoliters per hour (pl/hr)", "picoliters per minute (pl/min)", "picoliters per second (pl/sec)"] ("Flow Rate Units (1:ml/min)")
                                w883 = u16 0 items=["Infuse", "Withdraw"] ("Pump Direction (0:Infuse)")
                                n615 = local read "COMM Port:: Harvard Syringe Pump"() -> (w884:refnum<visa-resource-name>)
                                n616 = call <instrlib>:"Configure Flow Rate & Direction.vi"("VISA resource name"=w884, "Pump Direction (0:Infuse)"=w883, "Flow Rate (5.00)"=i8 2 ("Pump Address"), "Flow Rate Units (1:ml/min)"=w882) -> ("VISA resource name out"=w885:refnum<visa-resource-name>)  [unwired: 10 in, 1 out]
                                n617 = call <instrlib>:"Start Pump.vi"("Run Direction (0:Infuse)"=w886, "VISA resource name"=w885) -> ()  [unwired: 8 in, 2 out]
                                }
                                }
                                }
                                }
                                }
                                frame #2 {
                                n618 = Index Array(array=w889, index=2) -> (element=w890:dbl)
                                n619 = Greater Than 0?(x=w890) -> (x > 0?=w888:bool)
                                n620 = case shown="True" w888 {
                                tunnel: w892 -> [_ w894]
                                tunnel: w887 -> [_ w893]
                                frame False {
                                }
                                frame True {
                                n621 = call "PumpDispense.vi"("Flowrate(ul/min)"=w893, "Pump Address"="i", "Pump COMM Port"=w894) -> ()  [unwired: 7 in, 2 out]
                                }
                                }
                                }
                                frame #3 {
                                n622 = Index Array(array=w899, index=3) -> (element=w900:dbl)
                                n623 = Greater Than 0?(x=w900) -> (x > 0?=w898:bool)
                                n624 = case shown="True" w898 {
                                tunnel: w897 -> [_ w903]
                                tunnel: w896 -> [_ w902]
                                frame False {
                                }
                                frame True {
                                n625 = call "PumpDispense.vi"("Flowrate(ul/min)"=w902, "Pump Address"="e", "Pump COMM Port"=w903) -> ()  [unwired: 7 in, 2 out]
                                }
                                }
                                }
                                frame #4 {
                                n626 = Index Array(array=w908, index=4) -> (element=w909:dbl)
                                n627 = Greater Than 0?(x=w909) -> (x > 0?=w907:bool)
                                n628 = case shown="True" w907 {
                                tunnel: w906 -> [_ w912]
                                tunnel: w905 -> [_ w911]
                                frame False {
                                }
                                frame True {
                                n629 = call "PumpDispense.vi"("Flowrate(ul/min)"=w911, "Pump Address"="f", "Pump COMM Port"=w912) -> ()  [unwired: 7 in, 2 out]
                                }
                                }
                                }
                                frame #5 {
                                n630 = Index Array(array=w915, index=5) -> (element=w917:dbl)
                                n631 = Greater Than 0?(x=w917) -> (x > 0?=w916:bool)
                                n632 = case shown="True" w916 {
                                tunnel: w919 -> [_ w921]
                                tunnel: w914 -> [_ w920]
                                frame False {
                                }
                                frame True {
                                n633 = call "PumpDispense.vi"("Flowrate(ul/min)"=w920, "Pump Address"="h", "Pump COMM Port"=w921) -> ()  [unwired: 7 in, 2 out]
                                }
                                }
                                }
                                }
                                }
                                frame #1 {
                                n634 = while {
                                stop <- w928 stop-if-true
                                n635 = local read "Phase_Sensor_voltage"() -> (w923:dbl)
                                n636 = script code="organic_phase = 0;\nif start_phase_time \n   start_phase_timer = tic;\n   start_phase_time = 0;\nelse\n  %ignore phase sensor values\n  %if not(phase_sensor_val >2.9 && phase_sensor_val <3.8)\n    %    start_phase_timer = tic;\n   %end\n\n   end_phase_time =  toc(start_phase_timer )\n\n   if end_phase_time > 2\n       organic_phase = 1;\n       start_phase_time = 1;\n   end\n\nend"("phase_sensor_val"=w923) -> ("organic_phase"=w925:dbl)  [unwired: 1 in, 1 out]
                                n637 = local read "Stop"() -> (w927:bool)
                                n638 = Not Equal To 0?(x=w925) -> (x != 0?=w926:bool)
                                n639 = Or(x=w926, y=w927) -> (x .or. y?=w928:bool)
                                n640 = Wait (ms)(milliseconds to wait=u32 300) -> ()  [unwired: 1 out]
                                }
                                }
                                frame #2 {
                                n641 = local read "Stop"() -> (w931:bool)
                                n642 = Not(x=w931) -> (.not. x?=w930:bool)
                                n643 = local read "Sample Valve COMM::Port"() -> (w932:refnum<visa-resource-name>)
                                n644 = case shown="True" w930 {
                                tunnel: w932 -> [_ w934]
                                tunnel: w929 -> [_ w933]
                                frame False {
                                }
                                frame True {
                                n645 = flat-sequence {
                                tunnel: w933 -> [w936]
                                tunnel: w934 -> [w946]
                                frame #0 {
                                n646 = local read "Sample Valve COMM::Port"() -> (w935:refnum<visa-resource-name>)
                                n647 = flat-sequence {
                                tunnel: w938 -> [w943]
                                tunnel: [w943] -> w937
                                frame #0 {
                                n648 = Wait (ms)(milliseconds to wait=u32 500) -> ()  [unwired: 1 out]
                                }
                                }
                                n649 = call "NanoValve Load.vi"("VISA resource name"=w935) -> ()  [unwired: 10 in, 1 out]
                                n650 = call-poly <vilib>:"Digital Write.vi"("Output Value"=FALSE, "DO Channel"=u8 22, "LINX Resource"=w937) -> ()  [unwired: 7 in, 2 out]
                                n651 = call-poly <vilib>:"Digital Write.vi"("Output Value"=TRUE, "DO Channel"=u8 22, "LINX Resource"=w936) -> ("LINX Resource"=w938:T10)  [unwired: 7 in, 1 out]
                                }
                                frame #1 {
                                n652 = Wait (ms)(milliseconds to wait=u32 2000) -> ()  [unwired: 1 out]
                                }
                                frame #2 {
                                n653 = call "NanoValve Inject.vi"("VISA resource name"=w946) -> ()  [unwired: 10 in, 1 out]
                                }
                                }
                                }
                                }
                                }
                                frame #3 {
                                n654 = local read "Stop"() -> (w952:bool)
                                n655 = local read "Bay Parameters"() -> (w948:T2)
                                n656 = Unbundle By Name(w948) -> ("Hplc Wait time(min)"=w950:dbl)
                                n657 = Not(x=w952) -> (.not. x?=w951:bool)
                                n658 = case shown="True" w951 {
                                tunnel: w950 -> [_ w957]
                                tunnel: [errorcluster {"status"=FALSE, "code"=0, "source"=""} ("error out") w956] -> w949
                                tunnel: w948 -> [_ w955]
                                tunnel: w947 -> [_ w954]
                                frame False {
                                }
                                frame True {
                                n659 = flat-sequence {
                                tunnel: w957 -> [w959]
                                tunnel: w954 -> [w968]
                                tunnel: [w979] -> w956
                                tunnel: w955 -> [w978]
                                frame #0 {
                                # "Wait till for HPLC Method"
                                n660 = script code="start = tic;"() -> ("??"=w958:errorcluster)  [unwired: 1 in]
                                n661 = while {
                                tunnel: w959 -> [w961]
                                tunnel: w958 -> [w960]
                                stop <- w967 stop-if-true
                                n662 = Multiply(x=w961, y=60.0) -> (x*y=w962:dbl)
                                n663 = script code="end1 = toc(start);\nflush_time = 0;\nif end1 > hplc_wait_time\n   flush_time = 1;\nend"("??"=w960, "hplc_wait_time"=w962) -> ("flush_time"=w964:dbl)  [unwired: 1 out]
                                n664 = local read "Stop"() -> (w966:bool)
                                n665 = Not Equal To 0?(x=w964) -> (x != 0?=w965:bool)
                                n666 = Or(x=w965, y=w966) -> (x .or. y?=w967:bool)
                                }
                                }
                                frame #1 {
                                n667 = flat-sequence {
                                tunnel: w970 -> [w975]
                                tunnel: [w975] -> w969
                                frame #0 {
                                n668 = Wait (ms)(milliseconds to wait=u32 500) -> ()  [unwired: 1 out]
                                }
                                }
                                n669 = call-poly <vilib>:"Digital Write.vi"("Output Value"=FALSE, "DO Channel"=u8 24, "LINX Resource"=w968) -> ("LINX Resource"=w970:T10)  [unwired: 7 in, 1 out]
                                n670 = call-poly <vilib>:"Digital Write.vi"("Output Value"=TRUE, "DO Channel"=u8 24, "LINX Resource"=w969) -> ()  [unwired: 7 in, 2 out]
                                }
                                frame #2 {
                                n671 = Wait (ms)(milliseconds to wait=u32 30000) -> ()  [unwired: 1 out]
                                }
                                frame #3 {
                                n672 = Unbundle By Name(w978) -> ("hplc File Name"=w980:string)
                                n673 = call "hplc_analyze.vi"("File Path"=w980) -> ("error out"=w979:errorcluster)  [unwired: 10 in]
                                }
                                }
                                }
                                }
                                }
                                frame #4 {
                                n674 = Unbundle By Name(w982) -> ("status"=w983:bool)
                                n675 = case shown="False" w983 {
                                tunnel: w981 -> [_ w984]
                                frame False {
                                }
                                frame True {
                                n676 = while {
                                tunnel: w984 -> [w986]
                                stop <- w985 stop-if-true
                                w991 = "An error occured while trying to read HPLC data. " ("message")
                                n677 = local write "Error Message"(w991) -> ()
                                n678 = call <vilib>:"Three Button Dialog.vi"("Right Button Text (\"Cancel\")"="STOP EXPs" ("F button name (\"Cancel\")"), "Center Button Text (\"No\")"="REDO" ("T button name (\"OK\")"), "Left Button Text (\"Yes\")"="REREAD" ("T button name (\"OK\")"), "message"=w991) -> ("Which Button?"=w987:T19)  [unwired: 7 in]
                                n679 = case shown="\"Left Button\"" w987 {
                                tunnel: w986 -> [_ _ w998 _]
                                tunnel: [TRUE TRUE w997 w1000] -> w985
                                frame "Right Button" {
                                w992 = TRUE ("Setup Error")
                                n680 = local write "System Error"(w992) -> ()
                                n681 = local write "Setup Error"(w992) -> ()
                                n682 = script code="system_error = 1"() -> ()  [unwired: 1 in, 1 out]
                                n683 = local write "Stop"(w992) -> ()
                                }
                                frame "Center Button" {
                                n684 = script code="redo = true;\nopt_ctr = 1;\nCurrExp = CurrExp + 1;\nncall0 = ncall0 +1;\nif req_ctr == req_tot\n       opt_ctr = 3;\n  else\n     req_ctr = req_ctr +1;\nend"() -> ()  [unwired: 1 in, 1 out]
                                }
                                frame "Left Button" {
                                n685 = Unbundle By Name(w998) -> ("hplc File Name"=w999:string)
                                n686 = call "hplc_analyze.vi"("File Path"=w999) -> ("error out"=w995:errorcluster)  [unwired: 10 in]
                                n687 = Unbundle By Name(w995) -> ("status"=w996:bool)
                                n688 = Not(x=w996) -> (.not. x?=w997:bool)
                                }
                                frame "Window Close" {
                                w1000 = TRUE
                                n689 = local write "Setup Error"(w1000) -> ()
                                n690 = script code="system_error = 1"() -> ()  [unwired: 1 in, 1 out]
                                n691 = local write "Stop"(w1000) -> ()
                                }
                                }
                                }
                                }
                                }
                                }
                                frame #5 {
                                n692 = disable-structure shown="Disabled" {
                                frame Disabled {
                                n693 = flat-sequence {
                                tunnel: w1002 -> [w1007]
                                tunnel: [w1007] -> w1001
                                frame #0 {
                                n694 = Wait (ms)(milliseconds to wait=u32 500) -> ()  [unwired: 1 out]
                                }
                                }
                                n695 = call-poly <vilib>:"Digital Write.vi"("Output Value"=FALSE, "DO Channel"=u8 22) -> ("LINX Resource"=w1002:T10)  [unwired: 8 in, 1 out]
                                n696 = call-poly <vilib>:"Digital Write.vi"("Output Value"=TRUE, "DO Channel"=u8 22, "LINX Resource"=w1001) -> ()  [unwired: 7 in, 2 out]
                                }
                                frame Enabled {
                                }
                                }
                                }
                                }
                                }
                                }
                              }
                              frame #2 {
                                n697 = script code="C_measured =Conc;\nFvalues(end +1,:) = [Conc];"() -> ()  [unwired: 1 in, 1 out]
                                n698 = local write "HPLC Analysis"(TRUE ("HPLC Analysis")) -> ()
                              }
                            }
                          }
                          frame #4 {
                            n699 = local read "Stop"() -> (w1011:bool)
                            n700 = Not(x=w1011) -> (.not. x?=w1010:bool)
                            n701 = case shown="True" w1010 {
                              tunnel: [1.0 w1022] -> w1012
                              frame False {
                              }
                              frame True {
                                # "Save data to excel file"
                                n702 = local read "Bay Parameters"() -> (w1020:T2)
                                n703 = Unbundle By Name(w1020) -> ("Total Number of Experiments 2"=w1019:dbl)
                                n704 = script code="analyze_labview_results"("ncall"=w1019) -> ("terminate"=w1022:dbl, "ncall0"=w1021:dbl, "experiment_history"=w1017:dbl[][], "Pbest"=w1015:dbl[], "Tbest"=w1016:dbl[], "best_exp_num"=w1014:dbl)  [unwired: 1 in, 1 out]
                                n705 = local write "Flowrates(ul/min)_best"(w1015) -> ()
                                n706 = local write "temperature_best"(w1016) -> ()
                                n707 = local write "best_exp_num"(w1014) -> ()
                                n708 = local write "Current Experiment"(w1021) -> ()
                                n709 = local write "Total Number of Experiments"(w1019) -> ()
                                n710 = call-poly <vilib>:"Array To Matrix.vi"("Real 2D Array"=w1017) -> ("Real Matrix"=w1018:T18)
                                n711 = local write "experiment history"(w1018) -> ()
                              }
                            }
                          }
                          frame #5 {
                            n712 = local read "Num_exp_till_pause"() -> (w1024:i32)
                            n713 = Increment(x=w1024) -> (x+1=w1023:i32)
                            n714 = local write "Num_exp_till_pause"(w1023) -> ()
                          }
                          frame #6 {
                            # "Pause System"
                            n715 = local read "Bay Parameters"() -> (w1032:T2)
                            n716 = Unbundle By Name(w1032) -> ("Num_conditons_per_wait"=w1031:dbl)
                            n717 = local read "Num_exp_till_pause"() -> (w1030:i32)
                            n718 = Equal?(x=w1031, y=w1030) -> (x = y?=w1029:bool)
                            n719 = local read "Run_Stop_cluster"() -> (w1026:T7)
                            n720 = Unbundle By Name(w1026) -> ("Stop Run Button"=w1028:bool)
                            n721 = Or(x=w1028, y=w1029) -> (x .or. y?=w1027:bool)
                            n722 = case shown="True" w1027 {
                              tunnel: w1031 -> [w1035 _]
                              tunnel: w1030 -> [w1036 _]
                              tunnel: w1026 -> [_ w1038]
                              frame False {
                                n723 = Greater?(x=w1036, y=w1035) -> (0:w1034:bool)
                                n724 = case shown="True" w1034 {
                                frame False {
                                }
                                frame True {
                                n725 = local write "Num_exp_till_pause"(0 ("Num_exp_till_pause")) -> ()
                                }
                                }
                              }
                              frame True {
                                n726 = flat-sequence {
                                tunnel: w1038 -> [w1066]
                                frame #0 {
                                w1042 = string[] ["e", "f", "g", "h", "i", "j"]
                                # "Turn off pumps and stop controling temperature"
                                n727 = stacked-sequence {
                                frame #0 {
                                n728 = local write "Temperature Control 1"(FALSE ("Temperature Control 1")) -> ()
                                }
                                frame #1 {
                                n729 = local write "Temperature Control 2"(FALSE ("Temperature Control 2")) -> ()
                                }
                                frame #2 {
                                n730 = local write "Temperature Control 3"(FALSE ("Temperature Control 3")) -> ()
                                }
                                frame #3 {
                                n731 = local write "Temperature Control 4"(FALSE ("Temperature Control 4")) -> ()
                                }
                                frame #4 {
                                n732 = local write "Temperature Control 5"(FALSE ("Temperature Control 5")) -> ()
                                }
                                }
                                n733 = local read "COMM Port:: Harvard Syringe Pump"() -> (w1040:refnum<visa-resource-name>)
                                n734 = local read "Syringe_pump?"() -> (w1039:bool)
                                n735 = local read "COMM Port :: Milligat Pumps"() -> (w1041:refnum<visa-resource-name>)
                                n736 = Array Size(array=w1042) -> (size(s)=w1043:i32)
                                n737 = case shown="True" w1039 {
                                tunnel: w1040 -> [_ w1051]
                                frame False {
                                }
                                frame True {
                                n738 = call <instrlib>:"Stop Pump.vi"("VISA resource name"=w1051) -> ()  [unwired: 9 in, 2 out]
                                }
                                }
                                n739 = for {
                                N: w1043 -> [_]
                                tunnel: w1042 -> [w1049] mode=indexing
                                tunnel: w1041 -> [w1050]
                                n740 = call "PumpStop.vi"("Pump Address"=w1049, "Pump COMM Port"=w1050) -> ()  [unwired: 9 in, 1 out]
                                }
                                }
                                frame #1 {
                                n741 = local read "Stop"() -> (w1054:bool)
                                n742 = Not(x=w1054) -> (.not. x?=w1053:bool)
                                n743 = case shown="True" w1053 {
                                frame False {
                                }
                                frame True {
                                n744 = while {
                                stop <- w1060 stop-if-true
                                # "Wait till user confirms system resume"
                                n745 = Two Button Dialog(message="System is currently paused. Refill Syringes, flush lines, then press OK to continue optimization.\nOr Redo to repeat condition ", 1:"REDO" ("F button name (\"Cancel\")"), 2:"OK" ("Left Button Text (\"Yes\")")) -> (T button?=w1056:bool)
                                n746 = case shown="False" w1056 {
                                tunnel: [TRUE TRUE] -> w1055
                                frame False {
                                n747 = script code="redo = true;"() -> ()  [unwired: 1 in, 1 out]
                                }
                                frame True {
                                }
                                }
                                n748 = local read "Stop"() -> (w1061:bool)
                                n749 = Or(x=w1055, y=w1061) -> (x .or. y?=w1060:bool)
                                }
                                }
                                }
                                n750 = local write "stop_xl_write"(TRUE ("stop_xl_write")) -> ()
                                }
                                frame #2 {
                                n751 = local write "Num_exp_till_pause"(0 ("Num_exp_till_pause")) -> ()
                                n752 = Bundle By Name(cluster=w1066, "Stop Run Button"=FALSE) -> (w1064:T7)
                                n753 = local write "Run_Stop_cluster"(w1064) -> ()
                                }
                                }
                              }
                            }
                          }
                          frame #7 {
                            w1069 = FALSE
                            n754 = local write "Equlibrating Temperature"(w1069) -> ()
                            n755 = local write "Calculate condition"(w1069) -> ()
                            n756 = local write "Flushing System"(w1069) -> ()
                            n757 = local write "HPLC Analysis"(w1069) -> ()
                            n758 = local write "stop_xl_write"(TRUE ("stop_xl_write")) -> ()
                          }
                        }
                        n759 = while {
                          stop <- w1096 stop-if-true
                          n760 = flat-sequence {
                            frame #0 {
                              n761 = script code="save_excel_time_data;"() -> ()  [unwired: 1 in, 1 out]
                            }
                            frame #1 {
                              n762 = Wait (ms)(milliseconds to wait=u32 30000) -> ()  [unwired: 1 out]
                            }
                          }
                          n763 = local read "Stop"() -> (w1097:bool)
                          n764 = local read "stop_xl_write"() -> (w1095:bool)
                          n765 = Or(x=w1095, y=w1097) -> (x .or. y?=w1096:bool)
                        }
                      }
                    }
                  }
                }
                n766 = Greater?(x=w597, y=w598) -> (0:w605:bool)
                n767 = Equal?(x=w603, y=1.0) -> (x = y?=w599:bool)
                n768 = local read "Stop"() -> (w606:bool)
                n769 = Or(x=w606, y=w605) -> (x .or. y?=w602:bool)
                n770 = Or(x=w599, y=w602) -> (x .or. y?=w601:bool)
                n771 = case shown="True" w599 {
                  frame False {
                  }
                  frame True {
                    w610 = u16 2 items=["System  Error", "System Running", "System Standby"] ("System Status")
                    n772 = local write "Stop"(TRUE ("Stop")) -> ()
                    n773 = local write "System Status"(w610) -> ()
                  }
                }
                "Optimization_loop_index" <- w607
              }
            }
          }
          n774 = while {
            tunnel: w585 -> [w1192]
            stop <- w1195 stop-if-true
            n775 = local read "Temperature Control 3"() -> (w1193:bool)
            n776 = local read "running?"() -> (w1191:bool)
            n777 = And(x=w1191, y=w1193) -> (x .and. y?=w1194:bool)
            n778 = case shown="True" w1194 {
              tunnel: w1192 -> [_ w1198]
              frame False {
                n779 = local write "Temp SS? 3"(TRUE) -> ()
              }
              frame True {
                # "Bay 3 Temperature Controller"
                n780 = local read "Temperature SP 3"() -> (w1199:dbl)
                n781 = local read "Temperature 3"() -> (w1202:dbl)
                n782 = Subtract(x=w1202, y=w1199) -> (x-y=w1211:dbl)
                n783 = Absolute Value(x=w1211) -> (abs(x)=w1213:dbl)
                n784 = Less Or Equal?(x=w1213, y=1.2) -> (x <= y?=w1210:bool)
                n785 = local write "Temp SS? 3"(w1210) -> ()
                n786 = local read "SSR Duration 3"() -> (w1220:dbl)
                n787 = call-poly <vilib>:"PID Online Autotuning.vi"("setpoint"=w1199, "manipulated variable"=w1220, "autotuning parameters"=T9 {"type of controller"=enum."PID", "relay cycles"=3, "relay amplitude"=1.0, "control specifications"=enum."Normal", "PV noise level"=0.1} ("Autotuning Parameters R1"), "process variable"=w1202, "PID gains in"=T8 {"Proportional gain Kc"=0.38538, "Integral time Ti (sec)"=0.524375, "Derivative time Ti (sec)"=0.12585} ("PID gains 2")) -> ("setpoint out"=w1218:dbl, "process variable out"=w1219:dbl, "PID gains out"=w1222:T17)  [unwired: 6 in, 2 out]
                n788 = Greater?(x=w1199, y=w1202) -> (0:w1209:bool)
                n789 = call <vilib>:"PID Autotuning (Temperature).vi"("desired temperature"=w1218, "measured temperature"=w1219, "PID gains in"=w1222, "output range"=cluster{"output high":dbl, "output low":dbl} {"output high"=3.0, "output low"=-1.0} ("Output range")) -> ("output"=w1215:dbl)  [unwired: 12 in, 3 out]
                n790 = Multiply(x=1000.0, y=w1215) -> (x*y=w1217:dbl)
                n791 = local write "SSR Duration 3"(w1215) -> ()
                n792 = Greater Than 0?(x=w1217) -> (x > 0?=w1208:bool)
                n793 = And(x=w1208, y=w1209) -> (x .and. y?=w1206:bool)
                n794 = Subtract(x=w1202, y=10.0) -> (x-y=w1204:dbl)
                n795 = Less?(x=w1204, y=w1199) -> (x < y?=w1207:bool)
                n796 = And(x=w1207, y=w1206) -> (x .and. y?=w1205:bool)
                n797 = case shown="True" w1205 {
                  tunnel: [errorcluster {"status"=FALSE, "code"=0, "source"=""} ("error out") w1234] -> _
                  tunnel: 4 -> [_ w1232]
                  tunnel: w1217 -> [w1228 w1233]
                  tunnel: [0.0 w1236] -> w1200
                  tunnel: w1199 -> [_ w1235]
                  tunnel: w1198 -> [_ w1231]
                  frame False {
                    n798 = Absolute Value(x=w1228) -> (abs(x)=w1229:dbl)
                    n799 = Wait (ms)(milliseconds to wait=w1229) -> ()  [unwired: 1 out]
                  }
                  frame True {
                    n800 = call "TurnOnRelayArduino.vi"("channel"=w1232, "duration"=w1233, "LINX Resource"=w1231) -> ("error out"=w1234:errorcluster)  [unwired: 7 in, 1 out]
                    n801 = script code="tempdiff3= SP3 - T3;\nif tempdiff3 > 10\n  if slope3 < .01\n     temp_check3 = temp_check3 + 1;\n  else\n      temp_check3 =0;\n  end\nend\n\nif temp_check3 > 9\n  temp_error3 = 1\nend"("SP3"=w1235) -> ("temp_error3"=w1236:dbl)  [unwired: 1 in, 1 out]
                  }
                }
                n802 = Not Equal To 0?(x=w1200) -> (x != 0?=w1201:bool)
                n803 = case shown="True" w1201 {
                  frame False {
                  }
                  frame True {
                    n804 = local write "Error Message"("Bay 3 Temperature Heating Error") -> ()
                  }
                }
                n805 = case shown="True" w1201 {
                  tunnel: w1201 -> [_ w1226]
                  frame False {
                  }
                  frame True {
                    n806 = local write "System Error"(w1226) -> ()
                    n807 = local write "Stop"(w1226) -> ()
                  }
                }
              }
            }
            n808 = Wait (ms)(milliseconds to wait=u32 400) -> ()  [unwired: 1 out]
            n809 = local read "Stop"() -> (w1195:bool)
          }
          n810 = while {
            tunnel: w585 -> [w1146]
            stop <- w1149 stop-if-true
            n811 = local read "running?"() -> (w1145:bool)
            n812 = Wait (ms)(milliseconds to wait=u32 400) -> ()  [unwired: 1 out]
            n813 = local read "Temperature Control 4"() -> (w1148:bool)
            n814 = And(x=w1145, y=w1148) -> (x .and. y?=w1147:bool)
            n815 = case shown="True" w1147 {
              tunnel: w1146 -> [_ w1152]
              frame False {
                n816 = local write "Temp SS? 4"(TRUE ("Temp SS? 4")) -> ()
              }
              frame True {
                # "Bay 4 Temperature Controller"
                n817 = local read "Temperature SP 4"() -> (w1155:dbl)
                n818 = local read "Temperature 4"() -> (w1158:dbl)
                n819 = Subtract(x=w1158, y=w1155) -> (x-y=w1165:dbl)
                n820 = Absolute Value(x=w1165) -> (abs(x)=w1167:dbl)
                n821 = Less Or Equal?(x=w1167, y=1.2) -> (x <= y?=w1164:bool)
                n822 = local write "Temp SS? 4"(w1164) -> ()
                n823 = local read "SSR Duration 4"() -> (w1168:dbl)
                n824 = call-poly <vilib>:"PID Online Autotuning.vi"("setpoint"=w1155, "manipulated variable"=w1168, "autotuning parameters"=T9 {"type of controller"=enum."PID", "relay cycles"=3, "relay amplitude"=1.0, "control specifications"=enum."Normal", "PV noise level"=0.1} ("Autotuning Parameters R1"), "process variable"=w1158, "PID gains in"=T8 {"Proportional gain Kc"=0.38538, "Integral time Ti (sec)"=0.524375, "Derivative time Ti (sec)"=0.12585} ("PID gains 2")) -> ("setpoint out"=w1170:dbl, "process variable out"=w1171:dbl, "PID gains out"=w1173:T17)  [unwired: 6 in, 2 out]
                n825 = call <vilib>:"PID Autotuning (Temperature).vi"("desired temperature"=w1170, "measured temperature"=w1171, "PID gains in"=w1173, "output range"=cluster{"output high":dbl, "output low":dbl} {"output high"=3.0, "output low"=-1.0} ("Output range")) -> ("output"=w1169:dbl)  [unwired: 12 in, 3 out]
                n826 = Subtract(x=w1158, y=10.0) -> (x-y=w1157:dbl)
                n827 = Less?(x=w1157, y=w1155) -> (x < y?=w1159:bool)
                n828 = Multiply(x=1000.0, y=w1169) -> (x*y=w1177:dbl)
                n829 = Greater?(x=w1155, y=w1158) -> (0:w1163:bool)
                n830 = Greater Than 0?(x=w1177) -> (x > 0?=w1162:bool)
                n831 = local write "SSR Duration 4"(w1169) -> ()
                n832 = And(x=w1162, y=w1163) -> (x .and. y?=w1161:bool)
                n833 = And(x=w1159, y=w1161) -> (x .and. y?=w1160:bool)
                n834 = case shown="True" w1160 {
                  tunnel: [errorcluster {"status"=FALSE, "code"=0, "source"=""} ("error out") w1188] -> _
                  tunnel: 5 -> [_ w1186]
                  tunnel: w1177 -> [w1182 w1187]
                  tunnel: w1155 -> [_ w1190]
                  tunnel: [0.0 w1189] -> w1154
                  tunnel: w1152 -> [_ w1185]
                  frame False {
                    n835 = Absolute Value(x=w1182) -> (abs(x)=w1183:dbl)
                    n836 = Wait (ms)(milliseconds to wait=w1183) -> ()  [unwired: 1 out]
                  }
                  frame True {
                    n837 = call "TurnOnRelayArduino.vi"("channel"=w1186, "duration"=w1187, "LINX Resource"=w1185) -> ("error out"=w1188:errorcluster)  [unwired: 7 in, 1 out]
                    n838 = script code="tempdiff4= SP4 - T4;\nif tempdiff4 > 10\n  if slope4 < .01\n     temp_check4 = temp_check4 + 1;\n  else\n      temp_check4 =0;\n  end\nend\n\nif temp_check4 > 9\n  temp_error4 = 1\nend"("SP4"=w1190) -> ("temp_error4"=w1189:dbl)  [unwired: 1 in, 1 out]
                  }
                }
                n839 = Not Equal To 0?(x=w1154) -> (x != 0?=w1153:bool)
                n840 = case shown="True" w1153 {
                  frame False {
                  }
                  frame True {
                    n841 = local write "Error Message"("Bay 4 Temperature Heating Error") -> ()
                  }
                }
                n842 = case shown="True" w1153 {
                  tunnel: w1153 -> [_ w1180]
                  frame False {
                  }
                  frame True {
                    n843 = local write "System Error"(w1180) -> ()
                    n844 = local write "Stop"(w1180) -> ()
                  }
                }
              }
            }
            n845 = local read "Stop"() -> (w1149:bool)
          }
          n846 = while {
            stop <- w590 stop-if-true
            n847 = script code="TempArr1=circshift(TempArr1,9);\nTempArr2=circshift(TempArr2,9);\nTempArr3=circshift(TempArr3,9);\nTempArr4=circshift(TempArr4,9);\nTempArr5=circshift(TempArr5,9);\n\nTempArr1(10)=T1;\nTempArr2(10)=T2;\nTempArr3(10)=T3;\nTempArr4(10)=T4;\nTempArr5(10)=T5;\n\n[slope1 temp] = polyfit([1,2,3,4,5,6,7,8,9,10]',TempArr1,1);\nslope1 = slope1(1);\n[slope2 temp] = polyfit([1,2,3,4,5,6,7,8,9,10]',TempArr2,1);\nslope2= slope2(1);\n[slope3 temp] = polyfit([1,2,3,4,5,6,7,8,9,10]',TempArr3,1);\nslope3 = slope3(1);\n[slope4 temp] = polyfit([1,2,3,4,5,6,7,8,9,10]',TempArr4,1);\nslope4 = slope4(1);\n[slope5 temp] = polyfit([1,2,3,4,5,6,7,8,9,10]',TempArr5,1);\nslope5 = slope5(1);"() -> ()  [unwired: 1 in, 1 out]
            n848 = Wait (ms)(milliseconds to wait=u32 600) -> ()  [unwired: 1 out]
            n849 = local read "Stop"() -> (w590:bool)
          }
          n850 = while {
            tunnel: w585 -> [w1100]
            stop <- w1103 stop-if-true
            n851 = local read "running?"() -> (w1099:bool)
            n852 = local read "Temperature Control 5"() -> (w1101:bool)
            n853 = And(x=w1099, y=w1101) -> (x .and. y?=w1102:bool)
            n854 = case shown="True" w1102 {
              tunnel: w1100 -> [_ w1106]
              frame False {
                n855 = local write "Temp SS? 5"(TRUE ("Temp SS? 5")) -> ()
              }
              frame True {
                # "Bay 5 Temperature Controller"
                n856 = local read "SSR Duration 5"() -> (w1122:dbl)
                n857 = local read "Temperature SP 5"() -> (w1108:dbl)
                n858 = local read "Temperature 5"() -> (w1111:dbl)
                n859 = Subtract(x=w1111, y=w1108) -> (x-y=w1119:dbl)
                n860 = Absolute Value(x=w1119) -> (abs(x)=w1121:dbl)
                n861 = Less Or Equal?(x=w1121, y=1.2) -> (x <= y?=w1118:bool)
                n862 = local write "Temp SS? 5"(w1118) -> ()
                n863 = call-poly <vilib>:"PID Online Autotuning.vi"("setpoint"=w1108, "manipulated variable"=w1122, "autotuning parameters"=T9 {"type of controller"=enum."PID", "relay cycles"=3, "relay amplitude"=1.0, "control specifications"=enum."Normal", "PV noise level"=0.1} ("Autotuning Parameters R1"), "process variable"=w1111, "PID gains in"=T8 {"Proportional gain Kc"=0.38538, "Integral time Ti (sec)"=0.524375, "Derivative time Ti (sec)"=0.12585} ("PID gains 2")) -> ("setpoint out"=w1124:dbl, "process variable out"=w1125:dbl, "PID gains out"=w1127:T17)  [unwired: 6 in, 2 out]
                n864 = call <vilib>:"PID Autotuning (Temperature).vi"("desired temperature"=w1124, "measured temperature"=w1125, "PID gains in"=w1127, "output range"=cluster{"output high":dbl, "output low":dbl} {"output high"=3.0, "output low"=-1.0} ("Output range")) -> ("output"=w1123:dbl)  [unwired: 12 in, 3 out]
                n865 = Multiply(x=1000.0, y=w1123) -> (x*y=w1131:dbl)
                n866 = Greater?(x=w1108, y=w1111) -> (0:w1116:bool)
                n867 = Greater Than 0?(x=w1131) -> (x > 0?=w1117:bool)
                n868 = local write "SSR Duration 5"(w1123) -> ()
                n869 = And(x=w1117, y=w1116) -> (x .and. y?=w1114:bool)
                n870 = Subtract(x=w1111, y=10.0) -> (x-y=w1112:dbl)
                n871 = Greater?(x=w1112, y=w1108) -> (0:w1115:bool)
                n872 = And(x=w1115, y=w1114) -> (x .and. y?=w1113:bool)
                n873 = case shown="True" w1113 {
                  tunnel: [errorcluster {"status"=FALSE, "code"=0, "source"=""} ("error out") w1142] -> _
                  tunnel: 6 -> [_ w1139]
                  tunnel: w1131 -> [w1136 w1140]
                  tunnel: [0.0 w1144] -> w1109
                  tunnel: w1108 -> [_ w1143]
                  tunnel: w1106 -> [_ w1141]
                  frame False {
                    n874 = Absolute Value(x=w1136) -> (abs(x)=w1137:dbl)
                    n875 = Wait (ms)(milliseconds to wait=w1137) -> ()  [unwired: 1 out]
                  }
                  frame True {
                    n876 = call "TurnOnRelayArduino.vi"("channel"=w1139, "duration"=w1140, "LINX Resource"=w1141) -> ("error out"=w1142:errorcluster)  [unwired: 7 in, 1 out]
                    n877 = script code="tempdiff5= SP5 - T5;\n\nif tempdiff5 > 10\n  if slope5 < .01\n     temp_check5 = temp_check5 + 1;\n  else\n      temp_check5 =0;\n  end\nend\n\nif temp_check5 >9\n  temp_error5 = 1\nend"("SP5"=w1143) -> ("temp_error5"=w1144:dbl)  [unwired: 1 in, 1 out]
                  }
                }
                n878 = Not Equal To 0?(x=w1109) -> (x != 0?=w1107:bool)
                n879 = case shown="True" w1107 {
                  frame False {
                  }
                  frame True {
                    n880 = local write "Error Message"("Bay 5 Temperature Heating Error") -> ()
                  }
                }
                n881 = case shown="True" w1107 {
                  tunnel: w1107 -> [_ w1134]
                  frame False {
                  }
                  frame True {
                    n882 = local write "Stop"(w1134) -> ()
                    n883 = local write "System Error"(w1134) -> ()
                  }
                }
              }
            }
            n884 = Wait (ms)(milliseconds to wait=u32 400) -> ()  [unwired: 1 out]
            n885 = local read "Stop"() -> (w1103:bool)
          }
        }
      }
      n886 = local read "IR Sensor Device"() -> (w61:T6)
      n887 = while {
        tunnel: errorcluster {"status"=FALSE, "code"=0, "source"=""} ("error out") -> [w132]
        tunnel: w61 -> [w151]
        stop <- w172 stop-if-true
        w129 = u8 7 items=["RAM IR raw  Ch1"=4, "RAM IR raw  Ch2"=5, "RAM T_A"=6, "RAM T_OBJ1"=7, "RAM T_OBJ2"=8, "EEPROM_To_max"=32, "EEPROM_To_min"=33, "EEPROM_PWM_CTRL"=34, "EEPROM_Ta_range"=35, "EEPROM_Emissivity_CorrCoeff"=36, "EEPROM_SMBus Address"=46, "EEPROM_ConfigReg"=37] ("Melexis_Cmmds")
        # "Bay 5 Temperature Read"
        # "Bay 4 Temperature Read"
        # "Bay 3 Temperature Read"
        # "Bay 2 Temperature Read"
        # "Bay 1 Temperature Read"
        n888 = local read "Stop"() -> (w172:bool)
        n889 = call "IRSensorNIRead.vi"("error in (no error)"=w132, "Melexis_Cmmds"=w129, "Address"=u8 1, "device reference"=w151) -> ("error out"=w154:errorcluster, "Temperature"=w152:dbl, "device reference out"=w150:T6)  [unwired: 5 in]
        n890 = local write "error out"(w154) -> ()
        n891 = Unbundle By Name(w154) -> ("status"=w153:bool)
        n892 = call-poly <vilib>:"PID Control Input Filter.vi"("input"=w152) -> ("output"=w165:dbl)  [unwired: 4 in]
        n893 = case shown="False" w153 {
          tunnel: w164 -> [w181 _]
          tunnel: [w181 w182] -> w169
          frame False {
            n894 = local write "Temperature 1"(w181) -> ()
          }
          frame True {
            n895 = local read "Temperature 1"() -> (w182:dbl)
          }
        }
        n896 = flat-sequence {
          tunnel: w165 -> [w195]
          tunnel: [w195] -> w164
          tunnel: w150 -> [w194]
          tunnel: [w194] -> w149
          frame #0 {
            n897 = Wait (ms)(milliseconds to wait=u32 100) -> ()  [unwired: 1 out]
          }
        }
        n898 = call "IRSensorNIRead.vi"("error in (no error)"=w132, "Melexis_Cmmds"=w129, "Address"=u8 2, "device reference"=w149) -> ("error out"=w141:errorcluster, "Temperature"=w142:dbl, "device reference out"=w144:T6)  [unwired: 5 in]
        n899 = local write "error out"(w141) -> ()
        n900 = Unbundle By Name(w141) -> ("status"=w146:bool)
        n901 = call-poly <vilib>:"PID Control Input Filter.vi"("input"=w142) -> ("output"=w163:dbl)  [unwired: 4 in]
        n902 = case shown="True" w146 {
          tunnel: w162 -> [w179 _]
          tunnel: [w179 w180] -> w168
          frame False {
            n903 = local write "Temperature 2"(w179) -> ()
          }
          frame True {
            n904 = local read "Temperature 2"() -> (w180:dbl)
          }
        }
        n905 = flat-sequence {
          tunnel: w163 -> [w192]
          tunnel: [w192] -> w162
          tunnel: w144 -> [w191]
          tunnel: [w191] -> w143
          frame #0 {
            n906 = Wait (ms)(milliseconds to wait=u32 100) -> ()  [unwired: 1 out]
          }
        }
        n907 = call "IRSensorNIRead.vi"("error in (no error)"=w132, "Melexis_Cmmds"=w129, "Address"=u8 3, "device reference"=w143) -> ("error out"=w134:errorcluster, "Temperature"=w140:dbl, "device reference out"=w139:T6)  [unwired: 5 in]
        n908 = local write "error out"(w134) -> ()
        n909 = Unbundle By Name(w134) -> ("status"=w135:bool)
        n910 = case shown="False" w135 {
          tunnel: w159 -> [w177 _]
          tunnel: [w177 w178] -> w161
          frame False {
            n911 = local write "Temperature 3"(w177) -> ()
          }
          frame True {
            n912 = local read "Temperature 3"() -> (w178:dbl)
          }
        }
        n913 = call-poly <vilib>:"PID Control Input Filter.vi"("input"=w140) -> ("output"=w160:dbl)  [unwired: 4 in]
        n914 = flat-sequence {
          tunnel: w160 -> [w189]
          tunnel: [w189] -> w159
          tunnel: w139 -> [w188]
          tunnel: [w188] -> w137
          frame #0 {
            n915 = Wait (ms)(milliseconds to wait=u32 100) -> ()  [unwired: 1 out]
          }
        }
        n916 = call "IRSensorNIRead.vi"("error in (no error)"=w132, "Melexis_Cmmds"=w129, "Address"=u8 4, "device reference"=w137) -> ("error out"=w124:errorcluster, "Temperature"=w136:dbl, "device reference out"=w131:T6)  [unwired: 5 in]
        n917 = local write "error out"(w124) -> ()
        n918 = Unbundle By Name(w124) -> ("status"=w126:bool)
        n919 = case shown="True" w126 {
          tunnel: w157 -> [w175 _]
          tunnel: [w175 w176] -> w167
          frame False {
            n920 = local write "Temperature 4"(w175) -> ()
          }
          frame True {
            n921 = local read "Temperature 4"() -> (w176:dbl)
          }
        }
        n922 = call-poly <vilib>:"PID Control Input Filter.vi"("input"=w136) -> ("output"=w158:dbl)  [unwired: 4 in]
        n923 = flat-sequence {
          tunnel: w158 -> [w186]
          tunnel: [w186] -> w157
          tunnel: w131 -> [w185]
          tunnel: [w185] -> w130
          frame #0 {
            n924 = Wait (ms)(milliseconds to wait=u32 100) -> ()  [unwired: 1 out]
          }
        }
        n925 = call "IRSensorNIRead.vi"("error in (no error)"=w132, "Melexis_Cmmds"=w129, "Address"=u8 5, "device reference"=w130) -> ("error out"=w127:errorcluster, "Temperature"=w128:dbl)  [unwired: 5 in, 1 out]
        n926 = local write "error out"(w127) -> ()
        n927 = flat-sequence {
          tunnel: w156 -> [w183]
          tunnel: [w183] -> w155
          frame #0 {
            n928 = Wait (ms)(milliseconds to wait=u32 100) -> ()  [unwired: 1 out]
          }
        }
        n929 = Unbundle By Name(w127) -> ("status"=w125:bool)
        n930 = call-poly <vilib>:"PID Control Input Filter.vi"("input"=w128) -> ("output"=w156:dbl)  [unwired: 4 in]
        n931 = local write "error out"(w132) -> ()
        n932 = Build Array(w169, w168, w161, w167, w155) -> (w171:dbl[])
        n933 = Array To Cluster(array=w171) -> (cluster=→"Teperature Chart":T3)
        n934 = case shown="False" w125 {
          tunnel: w155 -> [w173 _]
          tunnel: [w173 w174] -> w166
          frame False {
            n935 = local write "Temperature 5"(w173) -> ()
          }
          frame True {
            n936 = local read "Temperature 5"() -> (w174:dbl)
          }
        }
        n937 = script code="MATLAB script"("T1"=w169, "T2"=w168, "T3"=w161, "T4"=w167, "T5"=w166) -> ()  [unwired: 1 in, 1 out]
      }
      n938 = while {
        stop <- w87 stop-if-true
        n939 = local read "Pump setpoint(ul/min) 1"() -> (w90:dbl)
        n940 = local read "Pump setpoint(ul/min) 2"() -> (w86:dbl)
        n941 = local read "Pump setpoint(ul/min) 3"() -> (w85:dbl)
        n942 = local read "Pump setpoint(ul/min) 4"() -> (w84:dbl)
        n943 = local read "Pump setpoint(ul/min) 5"() -> (w83:dbl)
        n944 = local read "Pump setpoint(ul/min) 6"() -> (w82:dbl)
        n945 = Build Array(w90, w86, w85, w84, w83, w82) -> (w91:dbl[])
        n946 = Array To Cluster(array=w91) -> (cluster=→"Pump Setpoints Chart":T3)
        n947 = Wait (ms)(milliseconds to wait=u32 5000) -> ()  [unwired: 1 out]
        n948 = local read "Stop"() -> (w87:bool)
      }
      n949 = while {
        stop <- w69 stop-if-true
        n950 = local read "System Error"() -> (w68:bool)
        n951 = Wait (ms)(milliseconds to wait=u32 300) -> ()  [unwired: 1 out]
        n952 = case shown="True" w68 {
          tunnel: [w73 w74] -> w66
          frame False {
            w70 = u16 2 items=["System  Error", "System Running", "System Standby"] ("System Status")
            w71 = u16 1 items=["System  Error", "System Running", "System Standby"] ("System Status")
            n953 = local read "running?"() -> (w72:bool)
            n954 = Select(t=w71, s=w72, f=w70) -> (s? t:f=w73:u16)
          }
          frame True {
            w74 = u16 0 items=["System  Error", "System Running", "System Standby"] ("System Status")
          }
        }
        n955 = local read "Stop"() -> (w69:bool)
        n956 = local write "System Status"(w66) -> ()
      }
      n957 = while {
        tunnel: w60 -> [w75]
        stop <- w81 stop-if-true
        n958 = call-poly <vilib>:"Analog Read.vi"("Analog Channel"=u8 0, "LINX Resource"=w75) -> ("Voltage"=w76:dbl)  [unwired: 6 in, 3 out]
        "Phase_Sensor_voltage" <- w76
        n959 = Wait (ms)(milliseconds to wait=u32 300) -> ()  [unwired: 1 out]
        n960 = Build Array(w76) -> (w78:dbl[])
        n961 = Array To Cluster(array=w78) -> (cluster=→"Phase Sensor Chart":T3)
        n962 = local read "Stop"() -> (w81:bool)
      }
      n963 = while {
        tunnel: w60 -> [w94]
        stop <- w119 stop-if-true
        w101 = 270
        w95 = 600
        w96 = 600
        # "Read Pressure and Flowrate"
        n964 = local read "Stop"() -> (w119:bool)
        n965 = call-poly <vilib>:"Analog Read.vi"("AI Channel(s)"=i32[] [14, 15, 14, 15], "LINX Resource"=w94) -> ("Voltages"=w92:dbl[])  [unwired: 6 in, 3 out]
        n966 = Index Array(array=w92, index=1) -> (element=w115:dbl)
        n967 = Index Array(array=w92, index=0) -> (element=w116:dbl)
        n968 = call-poly <vilib>:"PID Control Input Filter.vi"("input"=w115) -> ("output"=w108:dbl)  [unwired: 4 in]
        n969 = call-poly <vilib>:"PID Control Input Filter.vi"("input"=w116) -> ("output"=w107:dbl)  [unwired: 4 in]
        n970 = Multiply(x=104.96 ("y"), y=w108) -> (x*y=w109:dbl)
        n971 = Multiply(x=104.96 ("y"), y=w107) -> (x*y=w112:dbl)
        n972 = Subtract(x=w109, y=24.077) -> (x-y=w99:dbl)
        n973 = Subtract(x=w112, y=24.077) -> (x-y=w100:dbl)
        n974 = Build Array(w96, w95) -> (w104:i32[])
        n975 = Array To Cluster(array=w104) -> (cluster=→"Flowrate Chart":T4)
        n976 = Build Array(w100, w99) -> (w105:dbl[])
        n977 = local write "Flowrate Sensor 1"(w96) -> ()
        n978 = local write "Flowrate Sensor 2"(w95) -> ()
        n979 = local write "Pressure 1"(w100) -> ()
        n980 = local write "Pressure 2"(w99) -> ()
        n981 = Array To Cluster(array=w105) -> (cluster=→"Pressure Chart":T3)
        n982 = Wait (ms)(milliseconds to wait=u32 500) -> ()  [unwired: 1 out]
        n983 = script code="MATLAB script"("F1"=w96, "F2"=w95, "Pres1"=w100, "Pres2"=w99) -> ()  [unwired: 1 in, 1 out]
        n984 = Greater?(x=w99, y=w101) -> (0:w97:bool)
        n985 = Greater?(x=w100, y=w101) -> (0:w98:bool)
        n986 = case shown="True" w98 {
          frame False {
          }
          frame True {
            w123 = TRUE ("Stop")
            n987 = local write "System Error"(w123) -> ()
            n988 = local write "Stop"(w123) -> ()
            n989 = local write "Error Message"("Pressure Sensor 1 readings above 250psi") -> ()
            n990 = script code="system_error = 1;"() -> ()  [unwired: 1 in, 1 out]
          }
        }
        n991 = case shown="False" w97 {
          frame False {
          }
          frame True {
            w121 = TRUE ("Stop")
            n992 = local write "System Error"(w121) -> ()
            n993 = local write "Error Message"("Pressure Sensor 2 readings above 250psi") -> ()
            n994 = local write "Stop"(w121) -> ()
            n995 = script code="system_error = 1;"() -> ()  [unwired: 1 in, 1 out]
          }
        }
      }
    }
    frame #3 {
      # "Save and close xml and excel file"
      n996 = script code="if exist('xl_file','var') & exist('xlApp','var')\n  xlWorkbook.SaveAs(xl_file);\n  xlWorkbook.Close;\n  xlApp.Quit;\n  xlApp.delete;\nend"() -> ()  [unwired: 1 in, 1 out]
    }
    frame #4 {
      w1340 = string[] ["e", "f", "g", "h", "i", "j"]
      # "End communication to hardware"
      n997 = local read "Syringe_pump?"() -> (w1338:bool)
      n998 = local read "COMM Port:: Harvard Syringe Pump"() -> (w1339:refnum<visa-resource-name>)
      n999 = local read "IR Sensor Device"() -> (w1337:T6)
      n1000 = local read "COMM Port :: Milligat Pumps"() -> (w1342:refnum<visa-resource-name>)
      n1001 = call <vilib>:"Close.vi"("LINX Resource"=w1336) -> ()  [unwired: 10 in, 1 out]
      n1002 = Array Size(array=w1340) -> (size(s)=w1341:i32)
      n1003 = case shown="True" w1338 {
        tunnel: w1339 -> [_ w1343]
        frame False {
        }
        frame True {
          n1004 = call <instrlib>:"Stop Pump.vi"("VISA resource name"=w1343) -> ()  [unwired: 9 in, 2 out]
        }
      }
      n1005 = for {
        N: w1341 -> [_]
        tunnel: w1340 -> [w1344] mode=indexing
        tunnel: w1342 -> [w1345]
        n1006 = call "PumpStop.vi"("Pump Address"=w1344, "Pump COMM Port"=w1345) -> ()  [unwired: 9 in, 1 out]
        n1007 = Wait (ms)(milliseconds to wait=u32 100) -> ()  [unwired: 1 out]
      }
      n1008 = call-poly <vilib>:"NI-845x Close Reference.vi"("device reference"=w1337) -> ()  [unwired: 10 in, 1 out]
    }
    frame #5 {
      # "Display Error Messages if necessary"
      n1009 = local read "Error Message"() -> (w1347:string)
      n1010 = One Button Dialog(message=w1347) -> ()  [unwired: 1 in, 1 out]
    }
  }
